vi "FFT_Plugin.vi"(8 "Panel Refs":T1, 9 "Abort VI":refnum<vi>, 10 "Centre VI":refnum<vi>, 11 "Data reference":refnum<vi>) -> ()   [LabVIEW 2016]
uses:
  FFT_Plugin_states.ctl
  <userlib>/Import Export/Excel/Excel.lvclass
  <vilib>/Utility/miscctls.llb/LVMenuShortCut.ctl
  <vilib>/Analysis/baseanly.llb/Mean (DBL).vi
  <userlib>/_OpenG.lib/file/file.llb/Strip Path Extension - String__ogtk.vi
  <vilib>/Analysis/0measdsp.llb/Scaled Time Domain Window (DBL).vi
  <vilib>/Analysis/NI_AALPro.lvlib
  <vilib>/Analysis/NI_AALBase.lvlib
panel:
  in  "Start":dbl=81.44796380090499 format="%#.2g"
  in  "End":dbl=411.76470588235304 format="%#.2g"
  in  "Select data subset manually":bool=TRUE
  in  "Data subset selection":enum32{"Automatic", "Manual"}(radio)
  out "Mean":bool caption="Displaying mean traces"
  in  "Write SD":bool=TRUE caption="Write mean +/-SD"
  in  "Live displays":string="These graphs are live! If you keep this window open, these displays will update as you interact with EMA."
  in  "Frequency display":u16(ring) items=["Log Power Spectrum (dB)", "Power Contribution (RMS)", "Cumulative Power (RMS)"]
  in  "ID":string caption="ID (e.g. name or identifier)"
  in  "Write to Excel":bool
  in  "Inspect":bool
  out "Modifed":cluster{"Time":dbl[], "Data":dbl[]}[](graph)=[{"Time"=[0.0, 4.524886877828055, 9.04977375565611, 13.574660633484164, 18.09954751131222, 22.624434389140276, 27.14932126696833, 31.674208144796385, 36.19909502262444, 40.72398190045249, 45.24886877828055, 49.773755656108605, 54.29864253393666, 58.82352941176472, 63.34841628959277, 67.87330316742083, 72.39819004524888, 76.92307692307693, 81.44796380090499, 85.97285067873305, 90.4977375565611, 95.02262443438916, 99.54751131221721, 104.07239819004526, 108.59728506787332, 113.12217194570138, 117.64705882352943, 122.17194570135749, 126.69683257918554, 131.2217194570136, 135.74660633484166, 140.2714932126697, 144.79638009049776, 149.32126696832583, 153.84615384615387, 158.37104072398193, 162.89592760180997, 167.42081447963804, 171.9457013574661, 176.47058823529414, 180.9954751131222, 185.52036199095025, 190.04524886877832, 194.57013574660638, 199.09502262443442, 203.6199095022625, 208.14479638009053, 212.6696832579186, 217.19457013574663, 221.7194570135747, 226.24434389140276, 230.7692307692308, 235.29411764705887, 239.8190045248869, 244.34389140271497, 248.86877828054304, 253.39366515837108, 257.9185520361991, 262.4434389140272, 266.96832579185525, 271.4932126696833, 276.0180995475114, 280.5429864253394, 285.06787330316746, 289.5927601809955, 294.1176470588236, 298.64253393665166, 303.16742081447967, 307.69230769230774, 312.2171945701358, 316.74208144796387, 321.26696832579194, 325.79185520361995, 330.316742081448, 334.8416289592761, 339.36651583710415, 343.8914027149322, 348.4162895927602, 352.9411764705883, 357.46606334841636, 361.9909502262444, 366.5158371040725, 371.0407239819005, 375.56561085972857, 380.09049773755663, 384.6153846153847, 389.14027149321277, 393.6651583710408, 398.19004524886884, 402.7149321266969, 407.239819004525], "Data"=[0.0, 0.003280547685165013, 0.01289743101562241, 0.02868204224767145, 0.050222095798970356, 0.07622469955534793, 0.10470955152397791, 0.1342620908128156, 0.16506775984322497, 0.1981449543929827, 0.23299766292964016, 0.2662105902390335, 0.2931956236396307, 0.3120584889037999, 0.3258530645330844, 0.3402639325632184, 0.3582301135138749, 0.3764639485856317, 0.3875725425413241, 0.3867580700353336, 0.3767675391078517, 0.3655424378583449, 0.3566337965451223, 0.3388605051396726, 0.282325947397805, 0.14043659443059134, -0.15309830161500587, -0.7030469105570372, -1.6831700852742941, -3.3565583997790314, -6.061772265078592, -10.164326953796436, -16.003914225529716, -23.87323017982634, -34.03144146976264, -46.71611513029193, -62.11103033240042, -80.26582156132996, -101.01544876912169, -123.95678679339927, -148.5001403443597, -173.95829594178113, -199.6215568703556, -224.7966262246939, -248.82566464690345, -271.1095742967033, -291.1362617725535, -308.49403938519396, -322.8603880880117, -333.98337936102394, -341.68028983850377, -345.8596552383632, -346.546630418038, -343.8850717975933, -338.1095786339015, -329.5058674917241, -318.3815784329008, -305.05447076485876, -289.84936776232786, -273.0938258521163, -255.11142903316968, -236.21699940196743, -216.71734765310532, -196.91518147857133, -177.11029181867295, -157.5955080943795, -138.64867636996055, -120.52337364656901, -103.43967106564978, -87.57696817655224, -73.06973510057142, -60.0057900058209, -48.42657074882919, -38.328959252234895, -29.66966154027166, -22.37336695008905, -16.34303372017211, -11.468139565226295, -7.628722188583611, -4.697185233485573, -2.5417035402001376, -1.0322996914069509, -0.047157913061021184, 0.5100193652993072, 0.6618519237579549, 0.7367772454439462, 0.5977863432535553, 0.40162429098039726, 0.17091171829364973, 0.04844407747172897, 0.00765893596057796]}, {"Time"=[0.0, 4.524886877828055, 9.04977375565611, 13.574660633484164, 18.09954751131222, 22.624434389140276, 27.14932126696833, 31.674208144796385, 36.19909502262444, 40.72398190045249, 45.24886877828055, 49.773755656108605, 54.29864253393666, 58.82352941176472, 63.34841628959277, 67.87330316742083, 72.39819004524888, 76.92307692307693, 81.44796380090499, 85.97285067873305, 90.4977375565611, 95.02262443438916, 99.54751131221721, 104.07239819004526, 108.59728506787332, 113.12217194570138, 117.64705882352943, 122.17194570135749, 126.69683257918554, 131.2217194570136, 135.74660633484166, 140.2714932126697, 144.79638009049776, 149.32126696832583, 153.84615384615387, 158.37104072398193, 162.89592760180997, 167.42081447963804, 171.9457013574661, 176.47058823529414, 180.9954751131222, 185.52036199095025, 190.04524886877832, 194.57013574660638, 199.09502262443442, 203.6199095022625, 208.14479638009053, 212.6696832579186, 217.19457013574663, 221.7194570135747, 226.24434389140276, 230.7692307692308, 235.29411764705887, 239.8190045248869, 244.34389140271497, 248.86877828054304, 253.39366515837108, 257.9185520361991, 262.4434389140272, 266.96832579185525, 271.4932126696833, 276.0180995475114, 280.5429864253394, 285.06787330316746, 289.5927601809955, 294.1176470588236, 298.64253393665166, 303.16742081447967, 307.69230769230774, 312.2171945701358, 316.74208144796387, 321.26696832579194, 325.79185520361995, 330.316742081448, 334.8416289592761, 339.36651583710415, 343.8914027149322, 348.4162895927602, 352.9411764705883, 357.46606334841636, 361.9909502262444, 366.5158371040725, 371.0407239819005, 375.56561085972857, 380.09049773755663, 384.6153846153847, 389.14027149321277, 393.6651583710408, 398.19004524886884, 402.7149321266969, 407.239819004525], "Data"=[0.0, 0.0054566161286313305, 0.021176274392851222, 0.046402845232125546, 0.08050972395189936, 0.12246222159496195, 0.1706819140406933, 0.22432346829111416, 0.2842011841463597, 0.3513995755629801, 0.4251048686364699, 0.5014115385742612, 0.5744881966537195, 0.6410198013858962, 0.704505663049861, 0.7729203870067999, 0.8512494069665132, 0.9386660099878618, 1.0317819864568873, 1.1292110414085503, 1.237548340841314, 1.3742350110685522, 1.5563946190062303, 1.781662888227669, 2.013644189539546, 2.1740526496725328, 2.1439449687993104, 1.767900080639427, 0.8400325835065379, -0.9217802670351624, -3.863215671370597, -8.278985381773719, -14.131849697352102, -21.08840503957136, -29.34363717387475, -39.26921136340486, -51.09341268563484, -64.93747332101653, -80.80596778673693, -98.56733824438274, -117.95609965186719, -138.59151554993912, -160.00109682961426, -181.6431484493508, -202.93206429597086, -223.27426115269574, -242.11506061810584, -258.98865795683525, -273.55015617332555, -285.5623040534244, -294.83721215873993, -301.1821976891091, -304.40286334025706, -304.3669529493593, -301.07335219612645, -294.66137882028096, -285.359847882708, -273.4386074364175, -259.20346206447476, -243.01532144426855, -225.29165508030886, -206.4747759908676, -186.99390218825508, -167.25173298757048, -147.63117115923248, -128.49865329528657, -110.19326767484668, -93.00794725153561, -77.17352880118644, -62.85211863155751, -50.1398760216452, -39.073629946225466, -29.63596174019649, -21.75778010787348, -15.324114670246239, -10.18854434827308, -6.192684132978607, -3.18164831793366, -1.0092853331371683, 0.46464487735675375, 1.3769279294274739, 1.8573609250385243, 2.0215250875237833, 1.9543461091327725, 1.5020356466489981, 1.323737337596271, 1.0470392431337219, 0.7219573232570705, 0.38893025356732835, 0.14539394038923847, 0.029094749320411922]}, {"Time"=[0.0, 4.524886877828055, 9.04977375565611, 13.574660633484164, 18.09954751131222, 22.624434389140276, 27.14932126696833, 31.674208144796385, 36.19909502262444, 40.72398190045249, 45.24886877828055, 49.773755656108605, 54.29864253393666, 58.82352941176472, 63.34841628959277, 67.87330316742083, 72.39819004524888, 76.92307692307693, 81.44796380090499, 85.97285067873305, 90.4977375565611, 95.02262443438916, 99.54751131221721, 104.07239819004526, 108.59728506787332, 113.12217194570138, 117.64705882352943, 122.17194570135749, 126.69683257918554, 131.2217194570136, 135.74660633484166, 140.2714932126697, 144.79638009049776, 149.32126696832583, 153.84615384615387, 158.37104072398193, 162.89592760180997, 167.42081447963804, 171.9457013574661, 176.47058823529414, 180.9954751131222, 185.52036199095025, 190.04524886877832, 194.57013574660638, 199.09502262443442, 203.6199095022625, 208.14479638009053, 212.6696832579186, 217.19457013574663, 221.7194570135747, 226.24434389140276, 230.7692307692308, 235.29411764705887, 239.8190045248869, 244.34389140271497, 248.86877828054304, 253.39366515837108, 257.9185520361991, 262.4434389140272, 266.96832579185525, 271.4932126696833, 276.0180995475114, 280.5429864253394, 285.06787330316746, 289.5927601809955, 294.1176470588236, 298.64253393665166, 303.16742081447967, 307.69230769230774, 312.2171945701358, 316.74208144796387, 321.26696832579194, 325.79185520361995, 330.316742081448, 334.8416289592761, 339.36651583710415, 343.8914027149322, 348.4162895927602, 352.9411764705883, 357.46606334841636, 361.9909502262444, 366.5158371040725, 371.0407239819005, 375.56561085972857, 380.09049773755663, 384.6153846153847, 389.14027149321277, 393.6651583710408, 398.19004524886884, 402.7149321266969, 407.239819004525], "Data"=[0.0, 0.0011044792416986951, 0.004618587638393602, 0.010961239263217359, 0.019934467646041367, 0.02998717751573392, 0.03873718900726252, 0.04420071333451705, 0.0459343355400902, 0.044890333222985246, 0.040890457222810414, 0.03100964190380573, 0.011903050625541855, -0.01690282357829643, -0.052799533983692234, -0.09239252188036301, -0.13478917993876346, -0.18573811281659838, -0.25663690137423906, -0.3556949013378831, -0.4840132626256104, -0.6431501353518624, -0.8431270259159858, -1.103941877948324, -1.4489922947439358, -1.8931794608113501, -2.450141572029322, -3.1739939017535015, -4.206372754055126, -5.7913365325229, -8.260328858786588, -12.049668525819156, -17.87597875370733, -26.658055320081328, -38.719245765650534, -54.163018897179, -73.12864797916599, -95.59416980164337, -121.22492975150645, -149.34623534241578, -179.0441810368522, -209.32507633362317, -239.24201691109693, -267.950104000037, -294.71926499783604, -318.94488744071083, -340.1574629270011, -357.9994208135527, -372.1706200026979, -382.4044546686235, -388.5233675182676, -390.5371127876173, -388.69039749581884, -383.4031906458273, -375.1458050716765, -364.35035616316725, -351.4033089830936, -336.6703340933, -320.49527346018095, -303.17233025996404, -284.9312029860305, -265.95922281306724, -246.44079311795556, -226.57862996957223, -206.5894124781134, -186.69236289347248, -167.1040850650744, -148.03880004160243, -129.70581333011313, -112.30181772154698, -95.99959417949765, -80.93795006541633, -67.2171797574619, -54.90013839659631, -44.01520841029709, -34.558189551905016, -26.493383307365608, -19.754630812518933, -14.248159044030054, -9.8590153443279, -6.460335009827748, -3.9219603078524257, -2.1158409136458256, -0.9343073785341579, -0.17833179913308825, 0.14981715329162126, 0.14853344337338872, 0.08129125870372385, -0.04710681698002889, -0.04850578544578052, -0.013776877399256001]}] caption="XY Graph"
  in  "Abort":bool=TRUE
  in  "Periodic extension (zero padding)":bool
  in  "Remove DC Component":bool
  in  "Apply window":bool=TRUE
  in  "Window":u16(ring)=1 items=["Rectangle", "Hanning", "Hamming", "Blackman-Harris", "Exact Blackman", "Blackman", "Flat Top", "4 Term B-Harris ", "7 Term B-Harris", "Low Sidelobe", "Blackman Nuttall", "Triangle", "Bartlett-Hanning", "Bohman", "Parzen", "Welch", "Kaiser", "Dolph-Chebyshev", "Gaussian"]
  in  "stop":bool=TRUE
  in  "Live data":cluster{dbl, dbl, "Impulses":dbl[][]}(graph)={0.0, 4.524886877828055, "Impulses"=[[1.410730292612453, 1.3768034370367894, 1.3548353514357787, 1.341757359189093, 1.3252268542692756, 1.2918927209333702, 1.23781873081185, 1.1721445111231026, 1.1099562251709596, 1.0599166586354007, 1.0172490394533225, 0.9686595339431536, 0.9047673910478693, 0.8288181580322441, 0.7544025685957787, 0.694320690605783, 0.6505827404540062, 0.6137999925050119, 0.571742484121512, 0.519863429471382, 0.46442129820892636, 0.4156426193698084, 0.3761013091270612, 0.33311079925207554, 0.25992068556340814, 0.12161862542107932, -0.1252316400992416, -0.5453137519834004, -1.2425542690526563, -2.366660512170925, -4.095965103495613, -6.603127826568753, -10.026682854478048, -14.467711625845375, -20.006989082761383, -26.71765968791203, -34.650952736880704, -43.79728933083065, -54.05109908114851, -65.20716298219895, -76.99269469879322, -89.11260780001447, -101.28231848622046, -113.23974163442473, -124.7470593418671, -135.59518498445283, -145.61151288418924, -154.66139432364216, -162.6386816612302, -169.4536979266029, -175.03058130417614, -179.31745237847906, -182.3000030507743, -184.00518252156053, -184.4905185408141, -183.8271266774419, -182.08728700462382, -179.3406685891595, -175.65520191995512, -171.09721676508144, -165.72994784425535, -159.61282346036108, -152.804250039799, -145.3672457276378, -137.37444300835176, -128.91027361336867, -120.07028157394262, -110.95869222566036, -101.68453089228515, -92.35751827130296, -83.08446010208225, -73.96594451991314, -65.0928968197739, -56.542432632023775, -48.37445417938233, -40.632336128292174, -33.34854321380435, -26.550598679863526, -20.261661506765652, -14.494964066015047, -9.248487689619074, -4.506937349962988, -0.2522570296729517, 3.4294956811031243, 5.778147017617445, 8.70977538890169, 10.131569294830525, 10.597791415646018, 7.995318248677886, 5.088900932820739, 3.214356371728213, 1.4314128213908817], [2.364341969813819, 2.2900712202609257, 2.2245023155686567, 2.170743580247381, 2.124436396241567, 2.0755483929849197, 2.01770771754292, 1.9584047923111045, 1.9110386779575452, 1.8797060218748745, 1.855973634456436, 1.8244843934756714, 1.7728033605066527, 1.702529717788376, 1.6310446015189317, 1.5771716174771009, 1.5459564986366559, 1.5304339022630353, 1.522072725122912, 1.5178365238247493, 1.5254599916191358, 1.5625836578011185, 1.6413532856314563, 1.7514320485671622, 1.8538422807040986, 1.8827378712669303, 1.7537081854795642, 1.3712601700239306, 0.6201310740437038, -0.6499338605382539, -2.610391134020305, -5.378339264237013, -8.853807453958103, -12.780045283497623, -17.251042072603628, -22.458661695090797, -28.504364179132295, -35.43332955585003, -43.23745946198392, -51.851105985309815, -61.15656151769813, -70.99547223516495, -81.18002034102021, -91.5014764479077, -101.73861407351457, -111.6704005080021, -121.09360769422771, -129.84220710857412, -137.79899427032026, -144.88621710119986, -151.034549457443, -156.15358303107433, -160.13037797728035, -162.85992421311624, -164.28158909283007, -164.38783024920167, -163.2016549976529, -160.7537911271449, -157.08309739913255, -152.2526003678371, -146.3579048093173, -139.51587757309167, -131.84668092020377, -123.46901638065522, -114.5091552863219, -105.10957295384713, -95.42778931381324, -85.62687785264612, -75.8640663935449, -66.28301727917503, -57.01190134479019, -48.1639845840505, -39.83537487539351, -32.09682287160172, -24.98497267821006, -18.50344472249384, -12.63639284811454, -7.366030658195303, -2.6806321266190096, 1.433839728680736, 5.010222790892419, 8.109088276495406, 10.813538617119217, 13.141504022534892, 13.11317906694486, 15.648494786805148, 17.745722641436604, 19.050523822150993, 18.194312156332213, 15.27318503082378, 12.21069001533261, 7.3082855694758475], [0.4571186154110868, 0.46353565381265327, 0.4851683873029008, 0.512771138130805, 0.5260173122969842, 0.5082370488818209, 0.4579297440807799, 0.3858842299351005, 0.30887377238437397, 0.24012729539592703, 0.17852444445020899, 0.11283467441063588, 0.03673142158908582, -0.04489340172388767, -0.1222394643273742, -0.18853023626553478, -0.24479101772864342, -0.30283391725301145, -0.3785877568798881, -0.47810966488198536, -0.596617395201283, -0.7312984190615017, -0.8891506673773341, -1.0852104500630113, -1.3340009095772822, -1.6395006204247715, -2.004171465678047, -2.4618876739907316, -3.1052396121490164, -4.083387163803597, -5.58153907297092, -7.827916388900492, -11.199558254997994, -16.15537796819313, -22.762936092919137, -30.97665768073326, -40.79754129462911, -52.16124910581127, -64.8647387003131, -78.56321997908809, -92.82882787988831, -107.22974336486399, -121.38461663142071, -134.97800682094174, -147.75550461021965, -159.51996946090355, -170.12941807415075, -179.4805815387102, -187.47836905214015, -194.02117875200594, -199.02661315090927, -202.4813217258838, -204.46962812426827, -205.1504408300048, -204.6994479887981, -203.26642310568212, -200.97291901159474, -197.9275460511741, -194.22730644077768, -189.9418331623258, -185.1019908791934, -179.7097693476305, -173.76181915939424, -167.26547507462038, -160.2397307303816, -152.7109742728902, -144.712773834072, -136.2905065986746, -127.5049953910254, -118.4320192634309, -109.1570188593743, -99.76790445577578, -90.35041876415428, -80.98804239244583, -71.76393568055461, -62.76122753409051, -54.060693579494156, -45.73516670153175, -37.842690886912294, -30.423767860710832, -23.507198170130565, -17.12296297642138, -11.318052676465122, -6.282512660328643, -1.5568850317099683, 1.7710559909982306, 2.517415948224447, 2.1450590091410415, -2.20367565897644, -5.095383165182303, -5.781977271876183, -4.445459926694085], [0.5023568318808596, 0.4893032590680133, 0.49512843757511926, 0.500047627047562, 0.48387712339247213, 0.4463428139727666, 0.4105470731967099, 0.40463061098914344, 0.4376463080092003, 0.4918853432629796, 0.5385413016613759, 0.5616941128357155, 0.5692138239041419, 0.5821157750397432, 0.6149119682566897, 0.6655257740297786, 0.7208605817914435, 0.7698018741854714, 0.8103861925510321, 0.8474898436816303, 0.887864780805265, 0.9375185517498736, 1.0001445273795566, 1.0738398057046237, 1.149548314048465, 1.2179439408484987, 1.285144372535588, 1.3833571315004367, 1.55999092462304, 1.8436470995521317, 2.2106634093212976, 2.5828681847113555, 2.8655582613049986, 3.0017191555559726, 3.003243389547119, 2.9394601145426895, 2.899301727675939, 2.960927470291303, 3.187483759635348, 3.6357361507565598, 4.35242738097167, 5.351830664232269, 6.594802226039589, 7.9950808295073745, 9.4553018038476, 10.907483107105017, 12.32874338057431, 13.725053926941623, 15.099607683510994, 16.430135556602362, 17.66711227556626, 18.749505584342824, 19.626001891778035, 20.269644324484567, 20.678235309300817, 20.861161720497595, 20.823903454212292, 20.565781901123675, 20.09654832301661, 19.45749107439412, 18.72273690523542, 17.971852691824232, 17.251893874532406, 16.561074428958364, 15.868972337133066, 15.154425182879812, 14.427593002881142, 13.718510695871757, 13.045049915207473, 12.391027427844957, 11.713505451661385, 10.973422679301992, 10.166330988933517, 9.33132231376839, 8.53068543424369, 7.812179601817312, 7.177734260878598, 6.582336612566129, 5.9675827457377215, 5.306315108243301, 4.622820187801937, 3.9689980802963487, 3.376119088371326, 2.8823122355666553, 2.2903695084639235, 1.74682508021205, 1.087631196240318, 0.6199203351200653, 0.2799378552104854, 0.16439572434565985, 0.0984395550677905, 0.13231348780272795], [1.2806770464228152, 1.2819836526066268, 1.3057566437960637, 1.3078837401439865, 1.2635371713360157, 1.188015892586324, 1.1197640828738749, 1.0930985125685955, 1.1147036889851334, 1.1591139554508967, 1.1955980114109348, 1.2084889615010135, 1.1996192567179116, 1.1922705220673417, 1.2097121688099948, 1.2472776797782872, 1.2959433980469712, 1.355528349106264, 1.4105906990562982, 1.4493738626633803, 1.4827087235283551, 1.5235075063052412, 1.58268412391006, 1.6682273812114417, 1.76940993451494, 1.8699579946172311, 1.9759712136701804, 2.120593404919596, 2.3439389358508866, 2.6634060822558356, 3.0593535489211616, 3.473113221158675, 3.8150646225118967, 4.011252980545241, 4.070742022765055, 4.104461153750526, 4.2504728044926585, 4.576307211048022, 5.10283115778458, 5.8772169708494, 6.96669915513311, 8.395206659253137, 10.102375743870343, 11.967375447685601, 13.869958419320628, 15.725982547852617, 17.492807941831806, 19.179160195859225, 20.82597706014503, 22.429034114548333, 23.8931934945146, 25.09384321384666, 25.964849305648727, 26.51429989736166, 26.783843727193812, 26.817608056436, 26.65181277982765, 26.30940823133898, 25.804911564823364, 25.145509892363634, 24.33126903352085, 23.393061077570334, 22.421743479829725, 21.50330731642481, 20.626636229942143, 19.718396527916962, 18.74988133125357, 17.76195064348292, 16.827954501857313, 15.991592772861058, 15.2000443824661, 14.361934988791564, 13.47627515294208, 12.61968455014931, 11.846212531594242, 11.158577412867583, 10.527352100572394, 9.922823291343615, 9.335625633440277, 8.742743856118311, 8.0981342384547, 7.387103058776486, 6.649124875775302, 5.929925072660412, 5.229415266600543, 4.553123721380457, 3.703916334369808, 2.9664692085587516, 2.100478303350439, 1.0767837594622454, 0.8247909324752697, 0.7200327482509221], [-0.275963382661096, -0.3033771344706002, -0.3154997686458252, -0.30778848604886244, -0.29578292455107147, -0.29533026464079076, -0.29866993648045503, -0.2838372905903087, -0.23941107296673275, -0.17534326892493757, -0.11851540808818284, -0.08510073582958244, -0.061191608909627715, -0.02803897198785532, 0.02011176770338463, 0.08377386828127009, 0.1457777655359157, 0.18407539926467886, 0.21018168604576604, 0.24560582469988013, 0.2930208380821747, 0.35152959719450594, 0.41760493084905337, 0.4794522301978057, 0.5296866935819898, 0.5659298870797661, 0.5943175314009956, 0.6461208580812772, 0.776042913395193, 1.0238881168484277, 1.3619732697214335, 1.6926231482640357, 1.9160519000981007, 1.9921853305667037, 1.9357447563291825, 1.7744590753348528, 1.5481306508592194, 1.345547729534585, 1.2721363614861152, 1.3942553306637193, 1.7381556068102295, 2.308454669211401, 3.0872287082088357, 4.022786211329148, 5.040645188374573, 6.088983666357419, 7.164678819316811, 8.27094765802402, 9.37323830687696, 10.431236998656392, 11.441031056617923, 12.405167954838989, 13.287154477907341, 14.024988751607474, 14.572626891407822, 14.90471538455919, 14.995994128596935, 14.822155570908368, 14.388185081209857, 13.769472256424608, 13.114204776949986, 12.55064430607813, 12.082044269235087, 11.618841541491916, 11.111308444323988, 10.590453837842663, 10.105304674508714, 9.675070748260595, 9.262145328557631, 8.790462082828856, 8.22696652085667, 7.58491036981242, 6.856386824924953, 6.042960077387468, 5.215158336893138, 4.465781790767041, 3.828116421184802, 3.241849933788643, 2.5995398580351656, 1.8698863603682905, 1.1475061371491733, 0.5508931018162122, 0.10311330096735061, -0.1653006015271017, -0.6486762496726959, -1.0594735609563568, -1.5286539418891716, -1.7266285383186208, -1.5406025929294682, -0.7479923107709258, -0.6279118223396888, -0.45540577264546617], [0.1428609168455076, 0.14009219140856577, 0.11947094183009842, 0.10077072367996759, 0.10664090057570925, 0.1408336768786598, 0.18290439134056327, 0.20532583194411785, 0.19704920610655483, 0.17131130147226892, 0.1509822095157714, 0.1472165016489006, 0.15162634039696785, 0.14726502462371371, 0.12541493294154754, 0.09187568505023, 0.059738087262853436, 0.03763662423540375, 0.024354767043458726, 0.011872031120744184, -0.00918999562797793, -0.0452084842455664, -0.09561082366349702, -0.1497420825160259, -0.1891829523968459, -0.19914511043679145, -0.18438773967785893, -0.17412197827471515, -0.2042001861453794, -0.28370161023986207, -0.3747421958073463, -0.41126283022121707, -0.3532835017017899, -0.2380282980415485, -0.18401709146102072, -0.3383244204315349, -0.8030823749571163, -1.5930376472087437, -2.6484391507481364, -3.88027583371108, -5.2058441553407535, -6.553143684831892, -7.848861818194611, -9.01821298931344, -10.00567137165893, -10.79874350413909, -11.430302235646876, -11.95285993523213, -12.400011764816897, -12.759417712509943, -12.972360283883038, -12.96031169842876, -12.664019458488333, -12.071631899296586, -11.216711005472934, -10.14751511736184, -8.893711046765965, -7.462892813463602, -5.872300712223161, -4.184494771149863, -2.5064055575799684, -0.9440319396179457, 0.45049034184902637, 1.6921303705819244, 2.825883972816616, 3.87539217302074, 4.82232194829527, 5.629306467522421, 6.279705590623783, 6.796762560700551, 7.229567603800389, 7.6216667224063706, 7.986642529547609, 8.304001897706291, 8.535683828129462, 8.652899248132748, 8.658862383256903, 8.591141998324726, 8.497475232866881, 8.400366725850619, 8.279505830654616, 8.090912186563397, 7.808832818723973, 7.241765629335075, 6.764355433821842, 6.380256170327707, 5.610727778846916, 4.487705481763241, 2.3698890985403973, 1.046250262014416, 0.42115130680965274, 0.0698224820121571], [0.7895528092077438, 0.7889645815842736, 0.7864982274026173, 0.7729337942321055, 0.7600503286681314, 0.7669180118298423, 0.7893386673117864, 0.8006965234119674, 0.7842792421592614, 0.7493836302729078, 0.7189433695337686, 0.7060017388053474, 0.70276193720043, 0.6950077931420253, 0.6718222239528342, 0.627505042151405, 0.5768263030203996, 0.5455471491014274, 0.534831905263048, 0.5224517112206513, 0.49008901261597826, 0.43575610802911896, 0.3724430942425503, 0.316782300810857, 0.2902199423782129, 0.3120135773721317, 0.3700048441619669, 0.42741629635065864, 0.4514998031343632, 0.4382643470086537, 0.4390392345620275, 0.5309452349275028, 0.7486940203525712, 1.0750380030480298, 1.4611155862724352, 1.813727417358169, 2.000364202769248, 1.9140182677827258, 1.537245321751846, 0.954703019325799, 0.29623030530770667, -0.3512896640963268, -0.9703807431636662, -1.5589288536235344, -2.084259572863407, -2.5012370465985505, -2.7939964423148, -2.9808859933857335, -3.0964144401108022, -3.1865081450918087, -3.287512379703312, -3.3729256937246923, -3.3334063465379735, -3.040229895146185, -2.439124577777161, -1.574064829191606, -0.5235420399304385, 0.6653420228090638, 1.9710431349929163, 3.3341480502154575, 4.625873721771791, 5.7140661618930295, 6.5669030810059645, 7.268357929590209, 7.922340404082234, 8.562022331023298, 9.146307556723766, 9.609889191511309, 9.938233958837124, 10.205346009285696, 10.503607392913068, 10.880846490462496, 11.349120062138814, 11.847728145359298, 12.248885237974134, 12.459822111756324, 12.473877235002584, 12.361579285203078, 12.228256884357315, 12.111771330098415, 11.943313468034535, 11.649768995915846, 11.23741208771981, 10.810655788857671, 10.350963760424722, 9.800349076558891, 9.259991702318938, 8.304543842410949, 5.751621749962787, 3.4052503349066274, 1.885089117525665, 0.5426199180611824], [-0.5038309755167286, -0.5087801987671421, -0.5475563437424205, -0.5713923468721704, -0.5467685275167128, -0.48525065807252277, -0.4235298846306599, -0.39004485952373164, -0.39018082994615166, -0.40676102732836994, -0.41697895050222583, -0.4115687355075463, -0.39950925640649426, -0.4004777438945979, -0.42099235806973906, -0.44375367205094496, -0.4573501284946927, -0.47027390063061997, -0.48612237117613055, -0.49870764897916287, -0.5084690038719342, -0.5261730765202518, -0.5636647415695444, -0.6162664658429088, -0.6685858471719047, -0.7103037982457145, -0.7387803235176847, -0.7756602529000889, -0.859900175425122, -1.005667567488378, -1.18852362617672, -1.3534708953699368, -1.455261023756151, -1.5510945991311267, -1.8291497691944765, -2.490376258221239, -3.6065289526834805, -5.100093562200213, -6.834123623248119, -8.715254686747958, -10.707918615989215, -12.754997705567458, -14.727342893225556, -16.477497125003346, -17.927083170454456, -19.09624996167963, -20.06660802897895, -20.924833877078527, -21.703609089522992, -22.33232727992808, -22.657208188062764, -22.547697703132826, -21.994632570438693, -21.103033903446985, -19.994297433168708, -18.720965405532073, -17.26388005360149, -15.591127649736269, -13.715644559439239, -11.703137592515183, -9.638684836931727, -7.602130041128921, -5.665922397307911, -3.88409718842636, -2.270572458449002, -0.8112379849818177, 0.4983363398667757, 1.6487237435335342, 2.6211772224104406, 3.388179112115406, 3.955527814687709, 4.362486954350246, 4.624164996956404, 4.760275650053283, 4.822482418284791, 4.8459763845091715, 4.843847531511221, 4.820704711446375, 4.7666935813764475, 4.688962121602822, 4.615698193274695, 4.532055377210948, 4.3802535497281365, 3.6728754698124786, 3.177747107218962, 2.9601632640965225, 1.9614638553748929, 0.6708671211155335, -1.0118435528819925, -1.3127498108777953, -1.0427865039063593, -0.4029749540368681], [0.8533007616422014, 0.8320714964959047, 0.8196882933654313, 0.8079448596831116, 0.7909464909994228, 0.7720577378667189, 0.7635056302479306, 0.777559929756277, 0.8159745504156796, 0.8669422250473191, 0.9125946222233504, 0.9415719339262932, 0.9566162500524569, 0.9705010485562443, 0.9950317781156892, 1.033071260791991, 1.0791888986124714, 1.126300875048726, 1.1704139113090224, 1.2104036620287582, 1.2464404189402403, 1.2806429666154864, 1.3188071312898992, 1.3688967345275418, 1.4365238639336193, 1.5232877289212883, 1.6330808615694297, 1.7822404386987416, 2.001960136635468, 2.323609122176582, 2.7516079794967765, 3.2414643864195596, 3.6992278552060047, 4.007043642180823, 4.063210441143857, 3.818699939609508, 3.297149449733941, 2.5943461384802746, 1.859343611972152, 1.2614315398989966, 0.9494176760733919, 1.0154878240495895, 1.4775969310388501, 2.2885387520450227, 3.366144675673136, 4.626767037284251, 6.0051738601788385, 7.4572974725508185, 8.954058207717338, 10.476302823265534, 12.012709504190957, 13.555493386738936, 15.09133859202418, 16.59397400886831, 18.026729814882497, 19.354622714624302, 20.555735639729008, 21.621514871912634, 22.548510483073205, 23.332552996011753, 23.97154289854723, 24.472005878131295, 24.848352635834072, 25.113026435485096, 25.26799987291367, 25.306985796617738, 25.22601964536895, 25.030210349184628, 24.72819210254418, 24.3203216008959, 23.794965876471103, 23.140429901127757, 22.364005693671263, 21.500484468712234, 20.599894865575504, 19.700989592717224, 18.809711522101438, 17.899971707920724, 16.936911686472836, 15.904629518153554, 14.81716083665625, 13.703923100751274, 12.583386221685391, 11.317970683867356, 10.00342705553732, 8.850639889857053, 7.148870567430042, 5.36440522728091, 2.7657810100007008, 1.2787409249801975, 0.5603658606604953, 0.25694201094766267], [1.5756044428356446, 1.5430067625100912, 1.5252045261135034, 1.5092660936195208, 1.4835766061817832, 1.4478712367684148, 1.4168706830915894, 1.413345866123949, 1.4446614641472526, 1.49352412873363, 1.536466401015578, 1.5598875127117107, 1.5651397159981455, 1.5679944669255153, 1.5841381298942583, 1.6143550927415997, 1.6538353290681425, 1.7025283705373409, 1.755045328634939, 1.8032435899676944, 1.8476868554787071, 1.8908487046295532, 1.9365519425045128, 1.9975252455999897, 2.083885944833346, 2.1926306019069823, 2.3226303850165424, 2.4929140255467996, 2.7385391000381527, 3.0887982428339598, 3.5526226280568594, 4.11670909190989, 4.743993660945112, 5.3761892288248205, 5.943019533553599, 6.369635184996055, 6.594108333229062, 6.604955076530372, 6.474899468154027, 6.351842132618369, 6.400966142676911, 6.744519893206698, 7.437302873617837, 8.466845374653317, 9.762592408548993, 11.219659404281234, 12.735241308194377, 14.240715961567727, 15.71365830661301, 17.16737184021246, 18.628258131124745, 20.1088018919615, 21.58160862283678, 22.97562649993662, 24.210350214230214, 25.244805687567602, 26.09479781317968, 26.80346860997333, 27.40494548219024, 27.90911231545381, 28.303126656279794, 28.588313487252584, 28.81694974004713, 29.037816850709437, 29.21783520920017, 29.28273964522523, 29.203479766937182, 29.007387928683162, 28.731646497562927, 28.373739765747175, 27.88610416625275, 27.226070296868453, 26.406161410113874, 25.495359035001943, 24.5752414096585, 23.690130134772676, 22.833212330921462, 21.967321157506376, 21.050768666311708, 20.057121515396126, 18.983215634368655, 17.839769830829805, 16.643097895977448, 15.585359402191163, 14.41353444519629, 13.039368118577533, 11.564001575813588, 9.833831106825002, 6.67662681422695, 4.198669954222929, 2.1125273214943396, 1.2679975953042555], [0.13099708044875813, 0.1211362304817184, 0.11417206061735918, 0.10662362574670248, 0.09831637581706232, 0.09624423896502321, 0.11014057740427174, 0.14177399338860497, 0.18728763668410653, 0.24036032136100816, 0.28872284343112276, 0.3232563551408757, 0.34809278410676814, 0.37300763018697347, 0.40592542633712025, 0.4517874288423822, 0.5045424681568003, 0.550073379560111, 0.5857824939831058, 0.6175637340898219, 0.6451939824017734, 0.6704372286014195, 0.7010623200752858, 0.7402682234550938, 0.7891617830338923, 0.853944855935594, 0.943531338122317, 1.0715668518506836, 1.2653811732327829, 1.5584200015192042, 1.9505933309366936, 2.3662196809292295, 2.6544620494668973, 2.637898055536825, 2.1834013487341153, 1.2677646942229615, 0.00019056623881974488, -1.416262799569823, -2.756212244209723, -3.828979052820376, -4.502130790530128, -4.713544245107519, -4.482109011540135, -3.889767870563272, -3.030303057202722, -1.9661253297127317, -0.7248935878367, 0.6738789835339114, 2.1944581088216673, 3.78523380631861, 5.397160877257166, 7.002184881516372, 8.60106856121158, 10.212321517800003, 11.84310941553478, 13.464439741681002, 15.016673466278334, 16.43956113385194, 17.69207548395617, 18.755993676569695, 19.639959140814668, 20.355698269010006, 20.879755531621015, 21.188236020260756, 21.31816453662717, 21.331231948010245, 21.24855952380072, 21.053032769686094, 20.724737707525435, 20.266903436044622, 19.703827586689457, 19.05478950538706, 18.321849977228652, 17.505609902422524, 16.624548321492508, 15.711849050661773, 14.786210713281415, 13.83262225833507, 12.823054706633965, 11.75213752091098, 10.651106038943842, 9.568076370672742, 8.523674547393334, 7.05058196554355, 5.593319665878351, 4.661911661136573, 2.733739559046496, 0.8949793477368191, -1.1450647942255476, -1.641188104262534, -0.9917956001733492, -0.75411357340893], [2.2825610735445365, 1.6193230987095557, -1.2849820096799227, -4.320985047234379, -5.381459413060144, -4.176678713666436, -2.2882677530372515, -1.4904682232865523, -2.082428596286533, -2.854711803833296, -2.5515901864208974, -1.2330459814903496, -0.1952032354127965, -0.6387397674322222, -2.4710664162134135, -4.373059705639674, -4.970109636560661, -3.9761352472064044, -2.358589667102657, -1.4915748039657968, -2.0240172303013564, -3.334905748584171, -3.943125994157051, -2.59776279122075, 0.673805767698131, 4.420827434851322, 6.73737934298327, 6.66096186239298, 4.931261250610796, 3.446973885506109, 3.8746207505011148, 6.60264779986794, 10.847583718022422, 15.682044284208619, 20.964630804484898, 27.377257768501018, 35.75421884997374, 46.385669442385655, 58.79854550912392, 72.05157168374596, 85.24788809630584, 97.96181470436719, 110.36678021867398, 122.9565320416245, 135.96202963453283, 148.91112895943164, 160.82243042909846, 170.9642555285605, 179.44688998924005, 186.97120397453466, 193.91619456235878, 199.76175924005014, 203.59875464326404, 205.30018492540896, 206.0660271446944, 207.56317264519944, 210.3530823047164, 213.14734435130453, 213.71207601600776, 210.62498682422188, 204.28124128150628, 196.34608236643365, 188.3259176594273, 180.58796550691932, 172.50215221488756, 163.2571191835404, 152.49349289314904, 140.41009768840135, 127.57536538807628, 114.74636441393602, 102.67447441726486, 91.77285697713005, 81.86518265971054, 72.32320072168578, 62.60998857207962, 52.78974965415986, 43.45912169914968, 35.14887122859104, 27.82585939558083, 21.021946002791335, 14.435387239341427, 8.278363206656431, 2.9496253155434617, -1.3483760411605146, -4.160633670200097, -8.532165813134927, -11.373486399666636, -12.953226674643206, -10.198865386599625, -6.054972325489615, -3.886647748801941, -1.784995149317917], [31.6011387585613, 30.682176150333987, 17.13159058407684, 1.2606610189742007, 3.199298818738791, 8.431102090258182, 11.584523356481265, 11.346477745042716, 5.412579330152584, 2.0426748197454945, 11.896811492467464, 19.795470556122773, 20.2512474096065, 12.198745989097235, 1.0932285970344608, 1.830844124150338, 2.1780985391629253, -0.18461438053893042, 0.6658550416306879, 2.8643870458147482, 1.1631486547555325, 0.8057697554662275, 0.920369029296829, 1.4006393504641963, 17.823018782793266, 37.64837695486858, 49.672791208536836, 47.67975390494491, 34.15004911799332, 18.02334692906269, 8.517823974998423, 10.287150265764708, 14.683787746237256, 19.099861478361877, 24.629592912147448, 32.857133591546486, 43.16485429408401, 55.077675595207964, 69.03638739879156, 84.41392008040003, 100.54709162702244, 116.76094032880908, 130.63564324377433, 142.12937699804502, 155.4485930268446, 170.1061977896586, 182.00801734225274, 193.2831591404493, 204.30183877060807, 210.38851372249607, 212.73377704600048, 219.33484458227548, 228.7608321437212, 233.5317756318039, 233.3692916663306, 232.57719789614282, 234.2125372684578, 236.8057562757666, 237.51493955512007, 234.02289398738714, 226.22074703613265, 218.6461915562746, 214.28521323115413, 209.9594073899002, 202.79028140235388, 192.68543931215274, 181.1818595335017, 169.38570205611688, 156.98426361922046, 144.4142980757566, 133.15400009887, 123.33111052541403, 113.9736356053802, 104.071275964053, 92.54805570898645, 79.45793385574865, 66.75233055443037, 56.29128406978212, 47.78336374406572, 39.90741667429724, 32.041662925717226, 24.35017614741126, 17.28310909513854, 11.465912730521428, 5.75214178300728, 1.230524599838514, -1.5725452100641437, -2.4307882394015685, 2.583141530894702, 6.245604974146939, 7.262335553144695, 5.654160758145034], [-27.03601661147223, -27.443529952914872, -19.701554603436684, -9.90263111344296, -13.962217644859079, -16.784459517591053, -16.16105886255577, -14.32741419161582, -9.577436522725652, -7.752098427412086, -16.99999186530926, -22.26156251910347, -20.641653880432095, -13.476225523961679, -6.035361429461288, -10.576963535429687, -12.118317812284246, -7.767656113873878, -5.383034375836002, -5.847536653746342, -5.211183115358246, -7.475581252634569, -8.806621017610931, -6.596164932905697, -16.475407247397005, -28.806722085165934, -36.1980325225703, -34.35783018015895, -24.287526616771725, -11.129399158050472, -0.7685824739961937, 2.9181453339711707, 7.011379689807589, 12.26422709005536, 17.299668696822348, 21.89738194545555, 28.343583405863466, 37.69366328956335, 48.560703619456284, 59.689223287091885, 69.94868456558925, 79.16268907992529, 90.09791719357362, 103.78368708520398, 116.47546624222105, 127.71606012920466, 139.63684351594418, 148.6453519166717, 154.59194120787203, 163.55389422657325, 175.09861207871708, 180.1886738978248, 178.4366771428069, 177.06859421901402, 178.7627626230582, 182.54914739425607, 186.493627340975, 189.48893242684244, 189.90921247689545, 187.22707966105662, 182.34173552687992, 174.0459731765927, 162.36662208770045, 151.21652362393843, 142.21402302742123, 133.82879905492806, 123.80512625279638, 111.4344933206858, 98.16646715693211, 85.07843075211545, 72.19494873565972, 60.21460342884606, 49.756729714040894, 40.575125479318565, 32.67192143517279, 26.12156545257108, 20.165912843868984, 14.006458387399963, 7.868355047095946, 2.1364753312854283, -3.170888447034372, -7.793449734098397, -11.383858464051617, -14.162664812842458, -14.073409123407474, -18.29485622610837, -21.17442758926913, -23.475665109884844, -22.98087230409395, -18.35554962512617, -15.035631050748577, -9.224151056780869], [-1.1981496477847582, -1.2478607091493559, -0.4972677927914925, 0.48005669892835245, 0.9959155512020954, 0.8227865344808531, 0.3538789450461943, 0.21056821192052508, 0.6542991333536923, 1.3525947019277265, 1.7145571624058944, 1.4472378634972867, 0.7832176592562639, 0.21888209791481628, 0.06259045619102394, 0.21990210358044887, 0.37377939670868654, 0.32318337599716396, 0.13181950738229678, -0.023701809606681723, -0.1005349069863002, -0.2592791153907109, -0.6689045311506439, -1.2444037388538263, -1.6224847522755697, -1.454289061786538, -0.791956150702996, -0.16828101558650402, -0.21104429464687258, -1.1239503660837502, -2.5201351335908626, -3.8036015331879853, -4.71483145078048, -5.452503521473123, -6.266936347855861, -7.04741605981341, -7.4503168125285235, -7.4282991364178725, -7.47044307479012, -8.129168111493136, -9.294778938885578, -10.115818528923805, -9.777712059859862, -8.33733920998134, -6.711530577346904, -5.8253823699826945, -5.854541726763927, -6.368658414108912, -7.075469803911694, -8.161600360867117, -9.774999340336551, -11.314683449277194, -11.551784176655634, -9.656484357429928, -6.092248938727362, -2.348018210481238, 0.33705660647427077, 2.008211503933337, 3.784312202061498, 6.665129866451432, 10.588256817764439, 14.569430928598218, 17.601892599428272, 19.35389261689661, 20.096018051074694, 20.176087972546274, 19.704184729852802, 18.67882384855385, 17.235221491711428, 15.67213657222401, 14.264144586499325, 13.099833463192951, 12.103687960677084, 11.145020390079699, 10.089057642000226, 8.807038222252451, 7.226045693098076, 5.42288717698219, 3.611021530002709, 1.9792553203757457, 0.5694983982567897, -0.6713215729586242, -1.7264661920179507, -2.427965711465797, -2.435216619568162, -2.579862187134526, -2.514457039007956, -2.782504686644563, -2.561875575189057, -2.0441084796839446, -1.362531396536606, -0.5852815158377919], [4.515475527764445, 6.6934451589817225, 7.487855134636235, 6.970868492876893, 6.0932797582553375, 4.693232105536136, 4.374886001478088, 4.906655003012542, 4.502308274827208, 4.861192620635503, 6.536753395251109, 6.431218471709848, 4.944409250799032, 3.9873332498503453, 3.547881596710193, 3.5159753484095813, 4.0484703294828135, 4.2843880036256206, 3.833157178924912, 3.0841172462458277, 3.0328961720500502, 3.4845787294685917, 3.1580437906241023, 2.3446760007881013, 2.7308431649357097, 4.3260954389714, 5.4002175065755464, 4.791733616623865, 3.866209229206044, 4.30135767132807, 3.3925116422451422, 0.7293104865251281, -0.7628452447355181, -0.5353460304838231, -1.5109182289741288, -2.523454248055545, -1.8944879891757145, -1.1856612719251869, -0.675360685773847, -0.5733749336038345, -1.4517410123473748, -1.648138146328554, -0.4822346477503121, 0.7582760046303143, 2.491907642879246, 4.145024303858277, 3.697943685123711, 4.5147229440079695, 7.856564242441199, 7.9332701405633745, 3.3639403855602126, 0.30460651211483736, 1.737309504643017, 3.585739958024046, 6.557559267408287, 11.18808503520422, 14.080574535276352, 15.803534784828983, 18.959245304263703, 22.518873615560267, 25.35184036589849, 27.86907241582484, 30.09452231290066, 31.279132519962367, 31.42319896628056, 31.34047886165137, 31.01513754798293, 29.49962527749096, 27.416848987979705, 26.702811012859506, 26.761549035428136, 25.941086451086015, 24.137639746007082, 21.989981926119412, 19.82339126178258, 17.637342339374648, 15.317203628361016, 13.22935703513324, 11.987902868641605, 11.041818254131226, 9.369272721674168, 6.757041032110883, 4.168978378348772, 3.342019175109911, 3.924034123236837, 3.7993869351913023, 3.398609874619339, 2.6344642392674915, 2.208737926594062, 2.1958484988039295, 2.350473055233414, 1.7286260384491916], [-6.911774823333961, -9.189166577280433, -8.48239072021922, -6.010755095020188, -4.101448655851146, -3.0476590365744305, -3.6671281113856997, -4.485518579171492, -3.193710008119824, -2.1560032167800505, -3.107639070439321, -3.5367427447152755, -3.3779739322865034, -3.549569054020713, -3.4227006843281456, -3.0761711412486834, -3.3009115360654406, -3.638021251631293, -3.5695181641603186, -3.131520865459191, -3.233965986022651, -4.003136960250013, -4.49585285292539, -4.833483478495754, -5.975812669486849, -7.234673562544476, -6.984129807981538, -5.128295647796873, -4.288297818499789, -6.549258403495569, -8.432781909426868, -8.3365135529011, -8.666817656825442, -10.369661012462423, -11.022954466737593, -11.571377871571276, -13.006145635881332, -13.670937000910559, -14.265525463806394, -15.68496128938244, -17.13781686542378, -18.583498911519058, -19.073189471969414, -17.432954424592996, -15.914968797573055, -15.795789043823666, -15.407027138651564, -17.252039772225793, -22.007503850264587, -24.25647086229761, -22.913939066233315, -22.933973410669225, -24.840877857954283, -22.898708672883902, -18.74205714486301, -15.884121456166694, -13.40646132232781, -11.787111776962309, -11.390620900140705, -9.188613882657402, -4.17532673036961, 1.2697894413715964, 5.109262885955882, 7.428652713830848, 8.76883713586883, 9.011697083441176, 8.39323191172267, 7.858022419616741, 7.053593995443153, 4.641462131588517, 1.7667401375705154, 0.2585804752998886, 0.0697361753470851, 0.30005885403998356, 0.3547240222178729, -0.023265894869743065, -0.865112242164864, -2.3835826811688596, -4.765859808636186, -7.083307613379734, -8.230275925160587, -8.09968417802813, -7.621910762384674, -8.197950598041505, -8.794467362373162, -8.959111309460354, -8.427523952635251, -8.199473612556616, -7.332489076972176, -6.284065458171819, -5.075535848306625, -2.899189070124775]]} caption="Impulse Trace"
  out "FFT":cluster{"Time":dbl[], "Data":dbl[]}[](graph)=[{"Time"=[0.0, 2.4285714285714284, 4.857142857142857, 7.285714285714285, 9.714285714285714, 12.142857142857142, 14.57142857142857, 17.0, 19.428571428571427, 21.857142857142854, 24.285714285714285, 26.71428571428571, 29.14285714285714, 31.57142857142857, 34.0, 36.42857142857142, 38.857142857142854, 41.285714285714285, 43.71428571428571, 46.14285714285714, 48.57142857142857, 50.99999999999999, 53.42857142857142, 55.857142857142854, 58.28571428571428, 60.71428571428571, 63.14285714285714, 65.57142857142857, 68.0, 70.42857142857142, 72.85714285714285, 75.28571428571428, 77.71428571428571, 80.14285714285714, 82.57142857142857, 85.0, 87.42857142857142, 89.85714285714285, 92.28571428571428, 94.71428571428571, 97.14285714285714, 99.57142857142857, 101.99999999999999, 104.42857142857142, 106.85714285714285, 109.28571428571428], "Data"=[-1.3284468668364369, 0.0, -5.385537504125523, -15.435463954020964, -28.20242502234497, -36.188627418479825, -46.821100679629254, -59.82657648738342, -60.12789326773007, -67.74033305448545, -67.43236104125887, -73.91497262179129, -75.66943487606963, -80.89084510184429, -84.78362519917926, -80.28925937165945, -84.83816971087651, -90.841165394456, -92.1008770459143, -93.12969892427525, -93.1239884835098, -93.59722396846385, -94.23913883751817, -95.03481857879969, -95.9652928205479, -97.02957823967398, -98.25272314777915, -99.47408973138023, -100.67995536129459, -101.75168970423206, -102.45169383683884, -102.67175862402809, -102.42667398970796, -101.89963744051411, -101.23341265726822, -100.54134369942744, -99.89589291671743, -99.32464398191397, -98.80941732312183, -98.3845599371269, -98.02216433701514, -97.7428271179752, -97.51070308349362, -97.34863812476058, -97.23662707082708, -97.18682747785813]}, {"Time"=[0.0, 2.4285714285714284, 4.857142857142857, 7.285714285714285, 9.714285714285714, 12.142857142857142, 14.57142857142857, 17.0, 19.428571428571427, 21.857142857142854, 24.285714285714285, 26.71428571428571, 29.14285714285714, 31.57142857142857, 34.0, 36.42857142857142, 38.857142857142854, 41.285714285714285, 43.71428571428571, 46.14285714285714, 48.57142857142857, 50.99999999999999, 53.42857142857142, 55.857142857142854, 58.28571428571428, 60.71428571428571, 63.14285714285714, 65.57142857142857, 68.0, 70.42857142857142, 72.85714285714285, 75.28571428571428, 77.71428571428571, 80.14285714285714, 82.57142857142857, 85.0, 87.42857142857142, 89.85714285714285, 92.28571428571428, 94.71428571428571, 97.14285714285714, 99.57142857142857, 101.99999999999999, 104.42857142857142, 106.85714285714285, 109.28571428571428], "Data"=[-1.5496705664320274, 0.0, -4.860110798865151, -14.282620783168522, -30.77984931740528, -46.152219964000075, -51.95422232313002, -54.37045094711479, -54.82263024205827, -56.939406462948014, -62.58803271330898, -69.04431891242457, -71.35646170319595, -69.31080988780718, -69.19769930168579, -73.75025679111238, -75.43436652276954, -78.22382878323597, -77.30505871462772, -77.4337955930445, -90.41534302179403, -79.06350388121508, -89.74022697118966, -82.77935421878425, -85.42023054868396, -88.81641833576619, -84.9722965929378, -98.16214696949471, -86.03666163274603, -95.08964128350334, -87.96710398201944, -90.71299662271774, -90.85530527000452, -89.12997346851843, -93.43042420377094, -89.05470640032148, -93.14289027030972, -89.91021718566888, -91.4989677958443, -91.22960482915276, -90.40701070072812, -92.2785530886493, -90.14914566743471, -92.27569921170073, -90.58063748214397, -91.45162598511088]}, {"Time"=[0.0, 2.4285714285714284, 4.857142857142857, 7.285714285714285, 9.714285714285714, 12.142857142857142, 14.57142857142857, 17.0, 19.428571428571427, 21.857142857142854, 24.285714285714285, 26.71428571428571, 29.14285714285714, 31.57142857142857, 34.0, 36.42857142857142, 38.857142857142854, 41.285714285714285, 43.71428571428571, 46.14285714285714, 48.57142857142857, 50.99999999999999, 53.42857142857142, 55.857142857142854, 58.28571428571428, 60.71428571428571, 63.14285714285714, 65.57142857142857, 68.0, 70.42857142857142, 72.85714285714285, 75.28571428571428, 77.71428571428571, 80.14285714285714, 82.57142857142857, 85.0, 87.42857142857142, 89.85714285714285, 92.28571428571428, 94.71428571428571, 97.14285714285714, 99.57142857142857, 101.99999999999999, 104.42857142857142, 106.85714285714285, 109.28571428571428], "Data"=[-1.1664218302869287, 0.0, -5.7999172506159695, -16.126850733058582, -25.046922928293256, -32.57940677094908, -43.62012841003624, -51.40538416440961, -52.82432008730757, -59.501501613398204, -67.88449467820614, -78.99659078715906, -69.41618652327307, -75.15196131993586, -74.0700380184418, -87.48910401615639, -84.19029121292672, -76.94576506118878, -81.41337096617008, -80.48057330313488, -87.55783937149215, -86.20008175730692, -86.99251041734308, -91.02851016920489, -90.14406054396127, -93.18013132602485, -92.85697631201948, -98.18672656053016, -93.43503954782327, -103.11159327800384, -95.36797475598117, -96.72344771486891, -101.65587037623936, -95.16626707924362, -106.5303029807485, -96.74734219532563, -99.93694557726481, -101.22780556340504, -98.42705017903822, -106.91053176743132, -100.06534004060818, -104.41194040340267, -105.50714131162829, -102.99558788371621, -114.4491400824021, -105.55212320416854]}] caption="XY Graph"
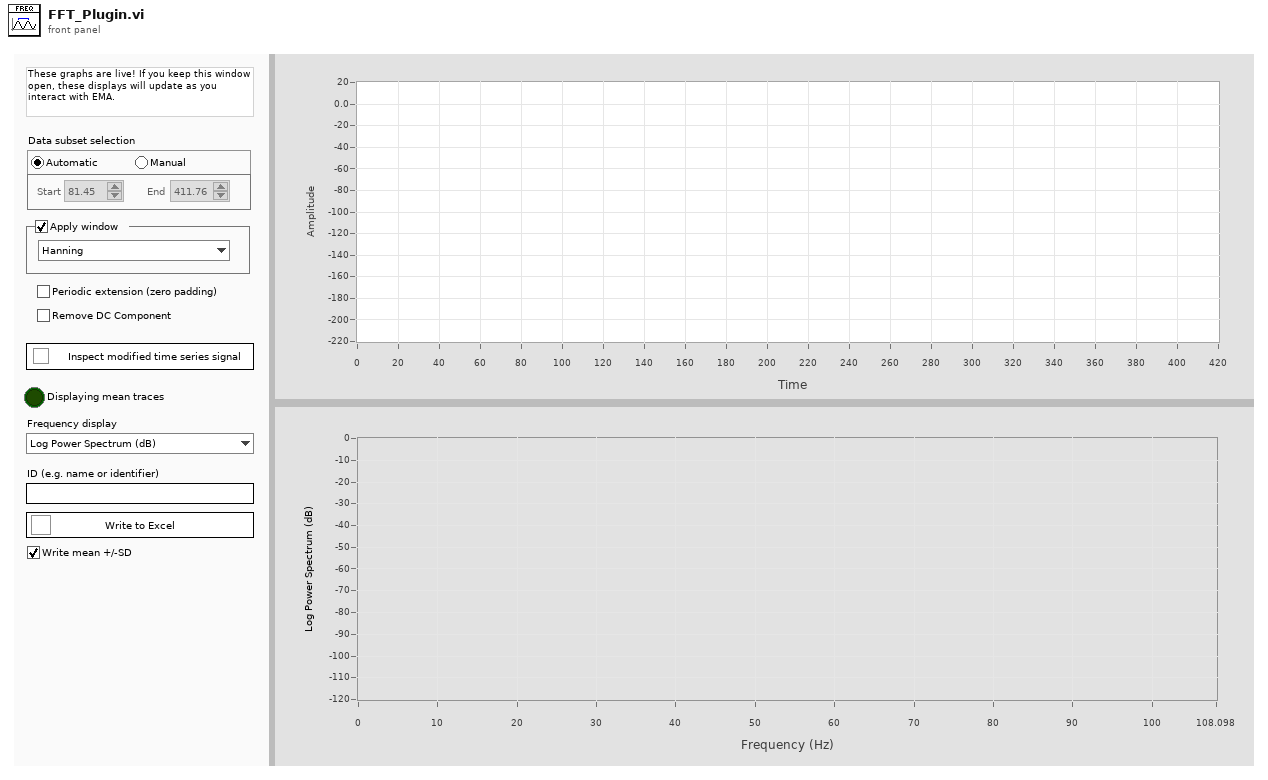
[diagram p1: front panel]
types:
  T1 = cluster{"Mean and STD":refnum<vi>, "Impulse dir":refnum<vi>, "Parameter Impuls Series":refnum<vi>, "Refresh":refnum<vi>}
  T2 = typedef "FFT_Plugin_states.ctl" = enum16{"Initialise", "Copy data", "Update cursors", "Perform FFT", "Launch inspection window", "Write to Excel", "Refresh", "Exit"}
  T3 = cluster{"Data header":string[], "Data":string[][], "Excel":refnum<class "Excel.lvclass">}
  T4 = typedef "LVMenuShortCut.ctl" = cluster{"Include Shift Key?":bool, "Include Ctrl Key?":bool, "Shortcut Key":string}
  T5 = cluster{"left":dbl, "top":dbl, "right":dbl, "bottom":dbl}
  T6 = cluster{"left":dbl, "top":dbl, "right":dbl, "bottom":dbl}[]
  T7 = cluster{"Horizontal":i32, "Vertical":i32, "Horizontal":i32, "Vertical":i32}[]
  T8 = enum32{"Invalid", "Standard", "Closed", "Hidden", "Minimized", "Maximized"}
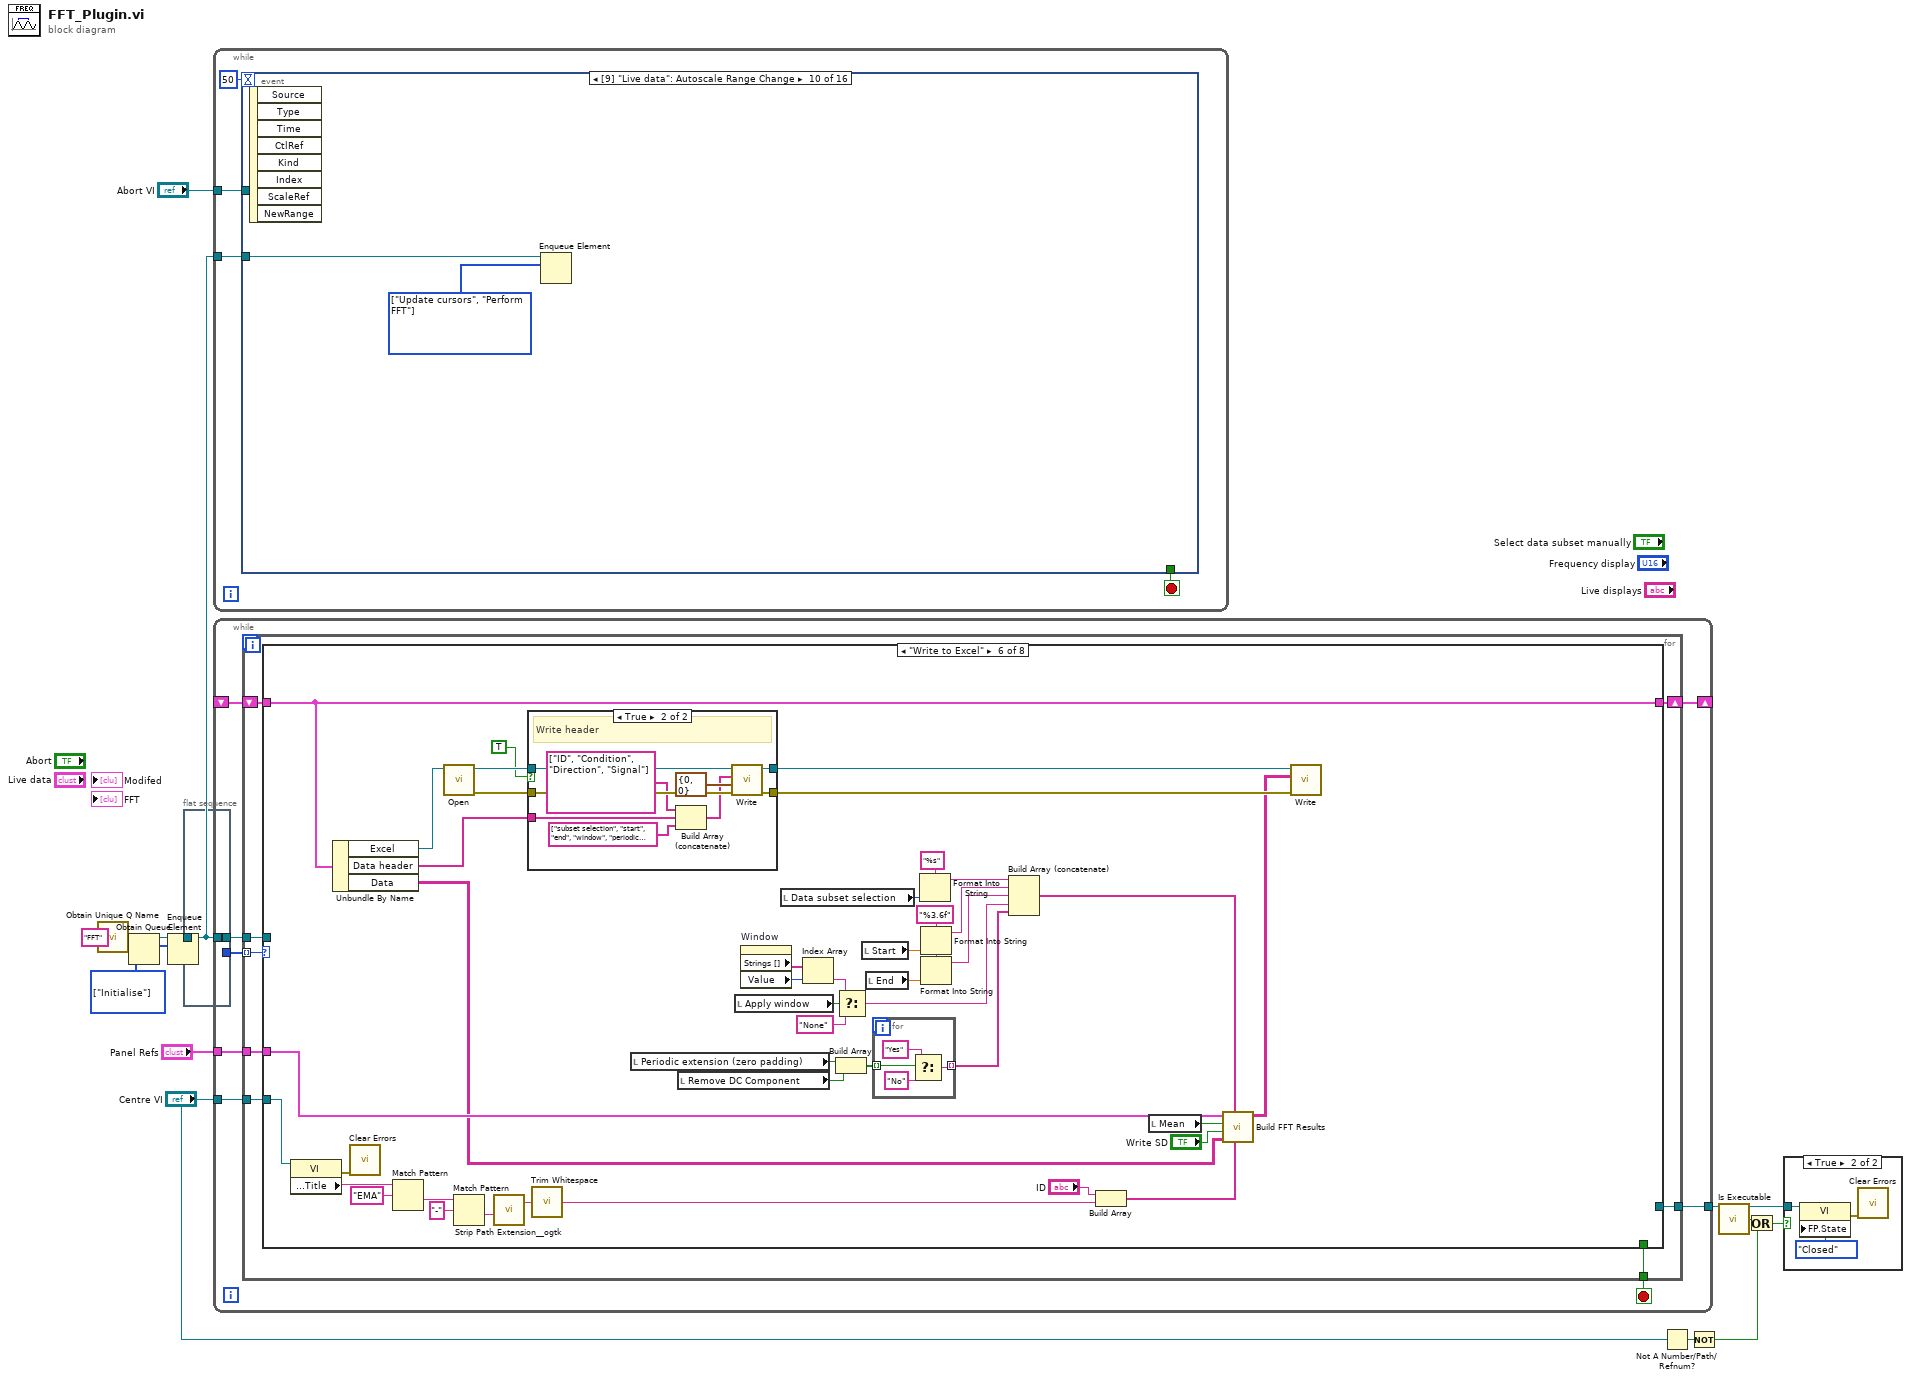
[diagram p0: block diagram]
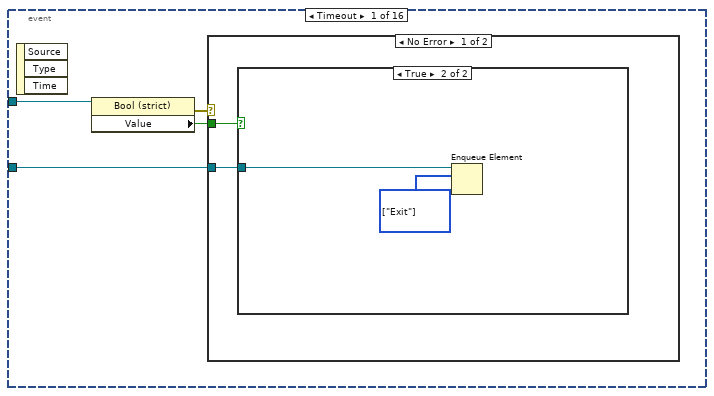
[diagram p2: hidden frame]
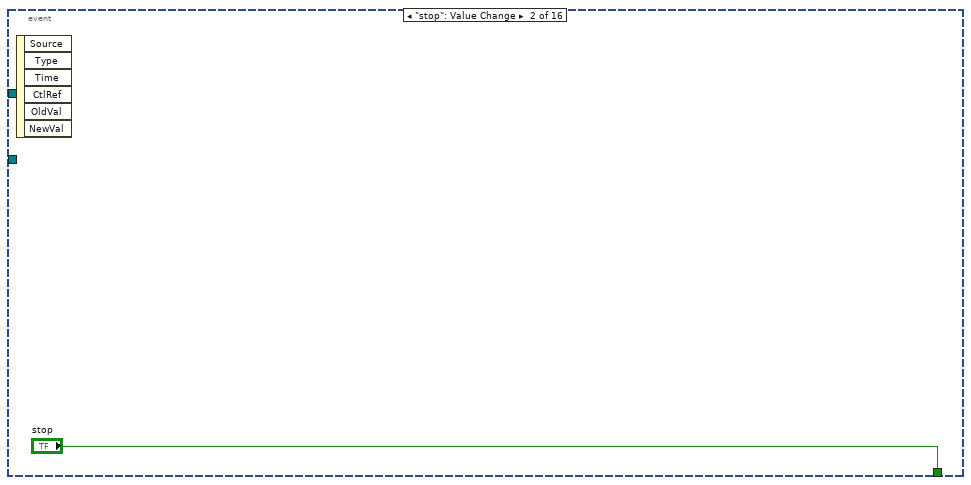
[diagram p5: hidden frame]
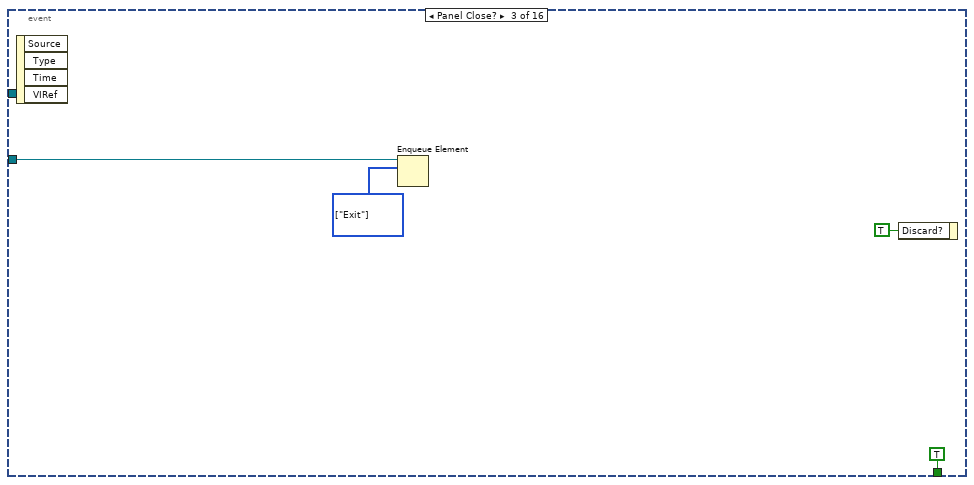
[diagram p6: hidden frame]
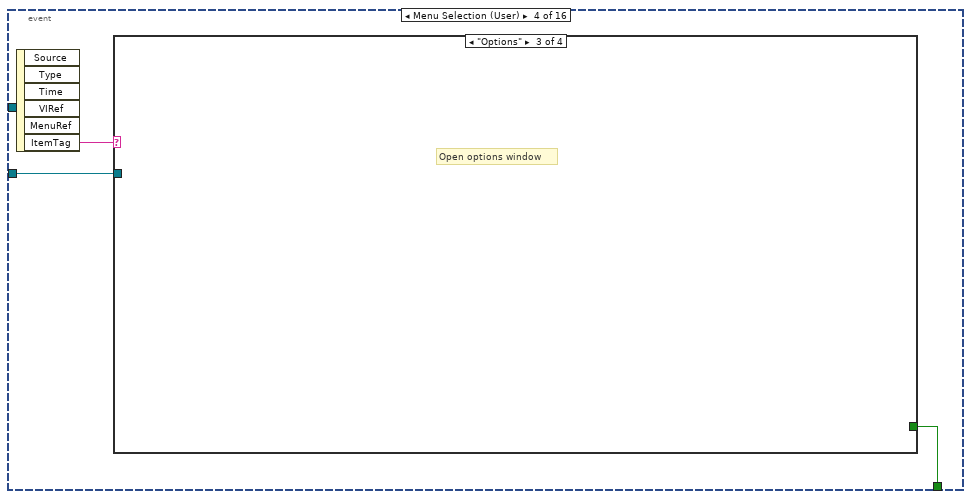
[diagram p7: hidden frame]
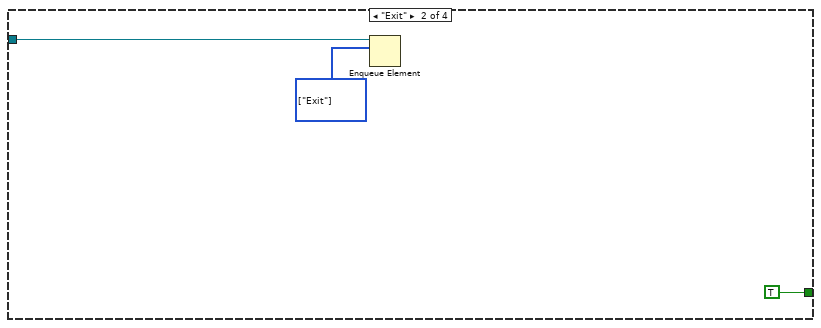
[diagram p9: hidden frame]
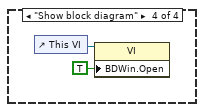
[diagram p10: hidden frame]
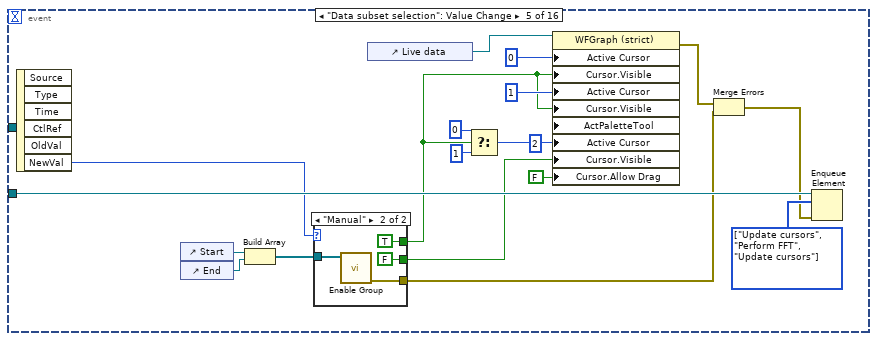
[diagram p11: hidden frame]
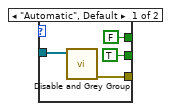
[diagram p12: hidden frame]
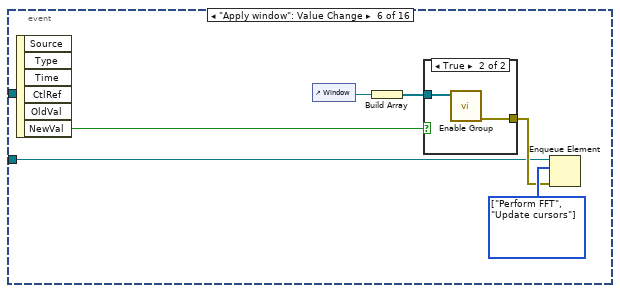
[diagram p13: hidden frame]
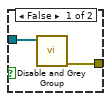
[diagram p14: hidden frame]
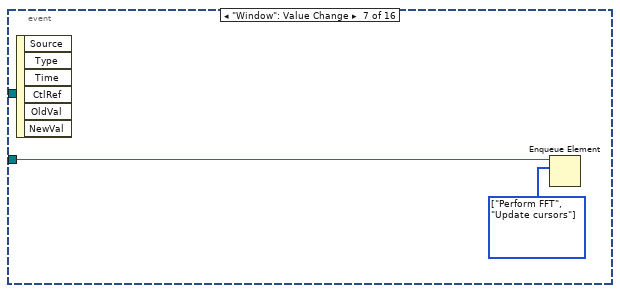
[diagram p15: hidden frame]
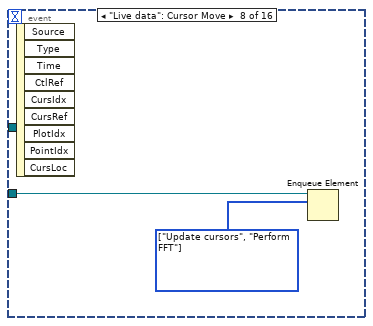
[diagram p16: hidden frame]
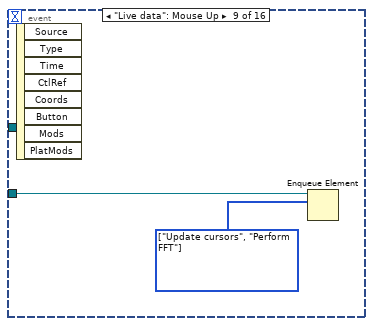
[diagram p17: hidden frame]
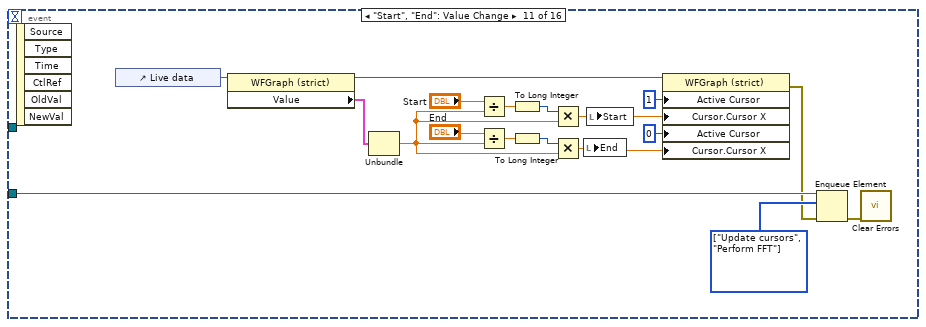
[diagram p18: hidden frame]
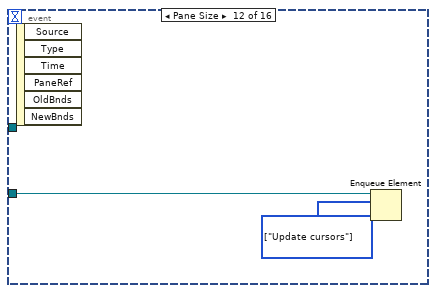
[diagram p19: hidden frame]
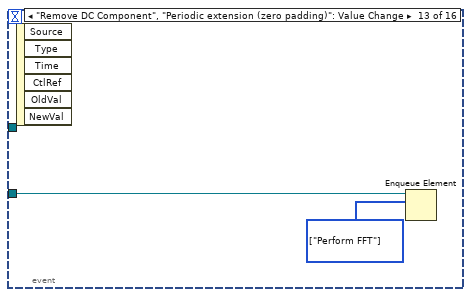
[diagram p20: hidden frame]
diagram:
  w10 = T2[] [enum."Initialise"] items=["Initialise", "Copy data", "Update cursors", "Perform FFT", "Launch inspection window", "Write to Excel", "Refresh", "Exit"]
  n1 = call <userlib>:"Obtain Unique Q Name.vi"("Queue"="FFT") -> ("Q Name"=w8:string)  [unwired: 4 in]
  n2 = Obtain Queue(name (unnamed)=w8, element data type=w10) -> (queue out=w9:refnum<queue>)  [unwired: 3 in, 2 out]
  n3 = Enqueue Element(queue=w9, element=w10) -> (queue out=w13:refnum<queue>)  [unwired: 2 in, 2 out]
  n4 = while {
    tunnel: w13 -> [w16]
    tunnel: "Abort VI" -> [w14]
    stop <- w17 stop-if-true
    n5 = event shown="[9] \"Live data\": Autoscale Range Change" {
      selector: _ -> [_ _ _ _ _ _ _ _ _ _ _ _ _ _ _ _]
      dyn-events: _ -> [_ _ _ _ _ _ _ _ _ _ _ _ _ _ _ _]
      timeout: 50 -> [_ _ _ _ _ _ _ _ _ _ _ _ _ _ _ _]
      tunnel: [_ "stop" TRUE w31 _ _ _ _ _ _ _ _ _ _ _ _] -> w17
      tunnel: w16 -> [w18 _ w29 w32 w52 w67 w76 w79 w81 w83 w91 w103 w105 w107 w109 w111]
      tunnel: w14 -> [w21 _ _ _ _ _ _ _ _ _ _ _ _ _ _ _]
      event Timeout {
        n6 = event-data() -> ()  [unwired: 1 in, 3 out]
        n7 = property class="Bool (strict)"(reference=w21) -> (error out=w19:errorcluster, "Value"=w20:bool)  [unwired: 1 in, 1 out]
        n8 = case shown="No Error" w19 {
          tunnel: w20 -> [w23 _]
          tunnel: w18 -> [w22 _]
          frame No Error {
            n9 = case shown="True" w23 {
              tunnel: w22 -> [_ w24]
              frame False {
              }
              frame True {
                w25 = T2[] [enum."Exit"] items=["Initialise", "Copy data", "Update cursors", "Perform FFT", "Launch inspection window", "Write to Excel", "Refresh", "Exit"]
                n10 = Enqueue Element(queue=w24, element=w25) -> ()  [unwired: 2 in, 3 out]
              }
            }
          }
          frame Error {
          }
        }
      }
      event "stop": Value Change {
        n11 = event-data() -> ()  [unwired: 1 in, 6 out]
      }
      event Panel Close? {
        w28 = T2[] [enum."Exit"] items=["Initialise", "Copy data", "Update cursors", "Perform FFT", "Launch inspection window", "Write to Excel", "Refresh", "Exit"]
        n12 = event-data() -> ()  [unwired: 1 in, 4 out]
        n13 = Enqueue Element(queue=w29, element=w28) -> ()  [unwired: 2 in, 3 out]
        n14 = event-data("Discard?"=TRUE) -> ()  [unwired: 1 in, 1 out]
      }
      event Menu Selection (User) {
        n15 = event-data() -> ("ItemTag"=w33:string)  [unwired: 1 in, 5 out]
        n16 = case shown="\"Options\"" w33 {
          tunnel: w32 -> [_ w36 _ _]
          tunnel: [_ TRUE _ _] -> w31
          frame Default {
          }
          frame "Exit" {
            w35 = T2[] [enum."Exit"] items=["Initialise", "Copy data", "Update cursors", "Perform FFT", "Launch inspection window", "Write to Excel", "Refresh", "Exit"]
            n17 = Enqueue Element(queue=w36, element=w35) -> ()  [unwired: 2 in, 3 out]
          }
          frame "Options" {
            # "Open options window"
          }
          frame "Show block diagram" {
            n18 = control-ref of="This VI"() -> (w38:refnum<vi>)
            n19 = property class="VI"(reference=w38, "BDWin.Open"=TRUE ("Block Diagram Window:Open")) -> ()  [unwired: 1 in, 2 out]
          }
        }
      }
      event "Data subset selection": Value Change {
        w51 = T2[] [enum."Update cursors", enum."Perform FFT", enum."Update cursors"] items=["Initialise", "Copy data", "Update cursors", "Perform FFT", "Launch inspection window", "Write to Excel", "Refresh", "Exit"]
        n20 = event-data() -> ("NewVal"=w43:enum32{"Automatic", "Manual"})  [unwired: 1 in, 5 out]
        n21 = control-ref of="Start"() -> (w54:refnum<vi>)
        n22 = control-ref of="End"() -> (w53:refnum<vi>)
        n23 = Build Array(w54, w53) -> (w55:refnum<vi>[])
        n24 = case shown="\"Manual\"" w43 {
          tunnel: w55 -> [w61 w65]
          tunnel: [w60 w64] -> w49
          tunnel: [FALSE TRUE] -> w42
          tunnel: [TRUE FALSE] -> w40
          frame "Automatic", Default {
            n25 = call <vilib>:"Disable and Grey Group.vi"("Group"=w61) -> ("error out"=w60:errorcluster)  [unwired: 9 in, 1 out]
          }
          frame "Manual" {
            n26 = call <vilib>:"Enable Group.vi"("Group"=w65) -> ("error out"=w64:errorcluster)  [unwired: 9 in, 1 out]
          }
        }
        n27 = control-ref of="Live data"() -> (w45:refnum<vi>)
        n28 = Select(t=0 ("Palette:Active Tool"), s=w42, f=1 ("Palette:Active Tool")) -> (s? t:f=w44:i32)
        n29 = property class="WFGraph (strict)"(reference=w45, "Active Cursor"=0, "Cursor.Visible"=w42, "Active Cursor"=1, "Cursor.Visible"=w42, "ActPaletteTool"=w44, "Active Cursor"=2, "Cursor.Visible"=w40, "Cursor.Allow Drag"=FALSE) -> (error out=w50:errorcluster)  [unwired: 1 in, 1 out]
        n30 = Merge Errors(w50, w49) -> (w48:errorcluster)
        n31 = Enqueue Element(queue=w52, element=w51, error in (no error)=w48) -> ()  [unwired: 1 in, 3 out]
      }
      event "Apply window": Value Change {
        w69 = T2[] [enum."Perform FFT", enum."Update cursors"] items=["Initialise", "Copy data", "Update cursors", "Perform FFT", "Launch inspection window", "Write to Excel", "Refresh", "Exit"]
        n32 = event-data() -> ("NewVal"=w71:bool)  [unwired: 1 in, 5 out]
        n33 = control-ref of="Window"() -> (w66:refnum<vi>)
        n34 = Build Array(w66) -> (w70:refnum<vi>[])
        n35 = case shown="True" w71 {
          tunnel: w70 -> [w73 w74]
          tunnel: [w72 w75] -> w68
          frame False {
            n36 = call <vilib>:"Disable and Grey Group.vi"("Group"=w73) -> ("error out"=w72:errorcluster)  [unwired: 9 in, 1 out]
          }
          frame True {
            n37 = call <vilib>:"Enable Group.vi"("Group"=w74) -> ("error out"=w75:errorcluster)  [unwired: 9 in, 1 out]
          }
        }
        n38 = Enqueue Element(queue=w67, element=w69, error in (no error)=w68) -> ()  [unwired: 1 in, 3 out]
      }
      event "Window": Value Change {
        w77 = T2[] [enum."Perform FFT", enum."Update cursors"] items=["Initialise", "Copy data", "Update cursors", "Perform FFT", "Launch inspection window", "Write to Excel", "Refresh", "Exit"]
        n39 = event-data() -> ()  [unwired: 1 in, 6 out]
        n40 = Enqueue Element(queue=w76, element=w77) -> ()  [unwired: 2 in, 3 out]
      }
      event "Live data": Cursor Move {
        w78 = T2[] [enum."Update cursors", enum."Perform FFT"] items=["Initialise", "Copy data", "Update cursors", "Perform FFT", "Launch inspection window", "Write to Excel", "Refresh", "Exit"]
        n41 = event-data() -> ()  [unwired: 1 in, 9 out]
        n42 = Enqueue Element(queue=w79, element=w78) -> ()  [unwired: 2 in, 3 out]
      }
      event "Live data": Mouse Up {
        w80 = T2[] [enum."Update cursors", enum."Perform FFT"] items=["Initialise", "Copy data", "Update cursors", "Perform FFT", "Launch inspection window", "Write to Excel", "Refresh", "Exit"]
        n43 = event-data() -> ()  [unwired: 1 in, 8 out]
        n44 = Enqueue Element(queue=w81, element=w80) -> ()  [unwired: 2 in, 3 out]
      }
      event "Live data": Autoscale Range Change {
        w82 = T2[] [enum."Update cursors", enum."Perform FFT"] items=["Initialise", "Copy data", "Update cursors", "Perform FFT", "Launch inspection window", "Write to Excel", "Refresh", "Exit"]
        n45 = event-data() -> ()  [unwired: 1 in, 8 out]
        n46 = Enqueue Element(queue=w83, element=w82) -> ()  [unwired: 2 in, 3 out]
      }
      event "Start", "End": Value Change {
        w92 = T2[] [enum."Update cursors", enum."Perform FFT"] items=["Initialise", "Copy data", "Update cursors", "Perform FFT", "Launch inspection window", "Write to Excel", "Refresh", "Exit"]
        n47 = event-data() -> ()  [unwired: 1 in, 6 out]
        n48 = control-ref of="Live data"() -> (w100:refnum<vi>)
        n49 = property class="WFGraph (strict)"(reference=w100) -> (reference out=w85:refnum<vi>, "Value"=w101:cluster{dbl, dbl, "Impulses":dbl[][]})  [unwired: 1 in, 1 out]
        n50 = Unbundle(w101) -> (w93:dbl)  [unwired: 2 out]
        n51 = Divide(x="Start", y=w93) -> (x/y=w99:dbl)
        n52 = Divide(x="End", y=w93) -> (x/y=w95:dbl)
        n53 = To Long Integer(number=w99) -> (32bit integer=w98:i32)
        n54 = To Long Integer(number=w95) -> (32bit integer=w96:i32)
        n55 = Multiply(x=w98, y=w93) -> (x*y=w89:dbl)
        n56 = Multiply(x=w96, y=w93) -> (x*y=w88:dbl)
        n57 = local write "End"(w88) -> ()
        n58 = local write "Start"(w89) -> ()
        n59 = property class="WFGraph (strict)"(reference=w85, "Active Cursor"=u32 1, "Cursor.Cursor X"=w89, "Active Cursor"=u32 0, "Cursor.Cursor X"=w88) -> (error out=w90:errorcluster)  [unwired: 1 in, 1 out]
        n60 = Enqueue Element(queue=w91, element=w92, error in (no error)=w90) -> (error out=w84:errorcluster)  [unwired: 1 in, 2 out]
        n61 = call <vilib>:"Clear Errors.vi"("error in (no error)"=w84) -> ()  [unwired: 5 in, 2 out]
      }
      event Pane Size {
        w102 = T2[] [enum."Update cursors"] items=["Initialise", "Copy data", "Update cursors", "Perform FFT", "Launch inspection window", "Write to Excel", "Refresh", "Exit"]
        n62 = event-data() -> ()  [unwired: 1 in, 6 out]
        n63 = Enqueue Element(queue=w103, element=w102) -> ()  [unwired: 2 in, 3 out]
      }
      event "Remove DC Component", "Periodic extension (zero padding)": Value Change {
        w104 = T2[] [enum."Perform FFT"] items=["Initialise", "Copy data", "Update cursors", "Perform FFT", "Launch inspection window", "Write to Excel", "Refresh", "Exit"]
        n64 = event-data() -> ()  [unwired: 1 in, 6 out]
        n65 = Enqueue Element(queue=w105, element=w104) -> ()  [unwired: 2 in, 3 out]
      }
      event "Inspect": Value Change {
        w106 = T2[] [enum."Launch inspection window"] items=["Initialise", "Copy data", "Update cursors", "Perform FFT", "Launch inspection window", "Write to Excel", "Refresh", "Exit"]
        n66 = event-data() -> ()  [unwired: 1 in, 6 out]
        n67 = Enqueue Element(queue=w107, element=w106) -> ()  [unwired: 2 in, 3 out]
      }
      event "Write to Excel": Value Change {
        w108 = T2[] [enum."Write to Excel"] items=["Initialise", "Copy data", "Update cursors", "Perform FFT", "Launch inspection window", "Write to Excel", "Refresh", "Exit"]
        n68 = event-data() -> ()  [unwired: 1 in, 6 out]
        n69 = Enqueue Element(queue=w109, element=w108) -> ()  [unwired: 2 in, 3 out]
      }
      event "Frequency display": Value Change {
        w110 = T2[] [enum."Perform FFT"] items=["Initialise", "Copy data", "Update cursors", "Perform FFT", "Launch inspection window", "Write to Excel", "Refresh", "Exit"]
        n70 = event-data() -> ()  [unwired: 1 in, 6 out]
        n71 = Enqueue Element(queue=w111, element=w110) -> ()  [unwired: 2 in, 3 out]
      }
    }
  }
  n72 = while {
    tunnel: w13 -> [w120]
    tunnel: [w116] -> w12
    shift-right: [w115] -> _
    shift-left: _ -> [w114]
    tunnel: "Centre VI" -> [w113]
    tunnel: "Panel Refs" -> [w112]
    stop <- w117 stop-if-true
    n73 = flat-sequence {
      tunnel: w120 -> [w127]
      tunnel: [w123] -> w118
      tunnel: [w126] -> w119
      frame #0 {
        w122 = T2[] [enum."Refresh"] items=["Initialise", "Copy data", "Update cursors", "Perform FFT", "Launch inspection window", "Write to Excel", "Refresh", "Exit"]
        n74 = Dequeue Element(queue=w127, timeout in ms (-1)=100) -> (queue out=w126:refnum<queue>, element=w121:T2[], timed out?=w124:bool)  [unwired: 1 in, 1 out]
        n75 = Select(t=w122, s=w124, f=w121) -> (s? t:f=w123:T2[])
      }
    }
    n76 = for {
      tunnel: w119 -> [w135]
      tunnel: w118 -> [w134] mode=indexing
      tunnel: [w133] -> w117
      tunnel: [w132] -> w116
      shift-right: [w131] -> w115
      shift-left: w114 -> [w130]
      tunnel: w113 -> [w129]
      tunnel: w112 -> [w128]
      n77 = case shown="\"Write to Excel\"" w134 {
        tunnel: w135 -> [w138 _ _ _ _ _ w448 _]
        tunnel: [_ _ _ _ _ _ _ TRUE] -> w133
        tunnel: [_ _ _ _ _ _ _ w457] -> w132
        tunnel: [w137 w214 w248 w264 w378 w421 w449 w455] -> w131
        tunnel: w130 -> [_ w214 w248 w265 w378 w421 w449 w455]
        tunnel: w129 -> [w136 w206 _ _ _ w413 _ _]
        tunnel: w128 -> [_ w194 _ _ _ w406 w443 _]
        frame "Initialise", Default {
          n78 = stacked-sequence {
            tunnel: w138 -> [_ _ _ w178]
            tunnel: [_ w146 _ _] -> w137
            tunnel: w136 -> [w139 _ _ _]
            frame #0 {
              # "Initialise"
              n79 = call <userlib>:"Centre window relative to caller.vi"("Enable (T)"=TRUE, "VI reference"=w139) -> ()  [unwired: 3 in, 1 out]
              n80 = local write "stop"(FALSE ("stop")) -> ()
              n81 = local write "Abort"(FALSE ("stop")) -> ()
              n82 = control-ref of="Live data"() -> (w142:refnum<vi>)
              n83 = property class="WFGraph (strict)"(reference=w142, "PlotImages.Front"=picture data[5B] ("Plot Images:Front")) -> ()  [unwired: 1 in, 2 out]
            }
            frame #1 {
              # "Build Program Cluster"
              n84 = call <userlib>:"Create.vi"() -> ("Excel out"=w145:refnum<class "Excel.lvclass">)  [unwired: 10 in, 1 out]
              n85 = Bundle By Name(cluster=T3 {"Data header"=["-3dB freq [0]", "-3dB freq [1]", "-6dB freq [0]", "-6dB freq [1]", "-9dB freq [0]", "-9dB freq [1]", "peak freq [0]", "peak power [0]", "peak freq [1]", "peak power [1]", "peak freq [2]", "peak power [2]"], "Data"=[], "Excel"=refnum} ("Program Cluster"), "Excel"=w145) -> (w146:T3)
            }
            frame #2 {
              # "Setup Menu"
              n86 = Current VI's Menubar() -> (w161:refnum<k9>)
              n87 = Delete Menu Items(9:w161) -> (3:w160:refnum<k9>)  [unwired: 3 in, 1 out]
              n88 = Insert Menu Items(7:string[] ["File", "Tools"] ("item tags"), 9:w160) -> (3:w159:refnum<k9>)  [unwired: 4 in, 2 out]
              n89 = Insert Menu Items(5:"File" ("menu tag"), 7:string[] ["Exit"] ("item tags"), 9:w159) -> (1:w152:string[], 3:w155:refnum<k9>)  [unwired: 3 in, 1 out]
              n90 = Insert Menu Items(5:"Tools" ("menu tag"), 7:string[] ["Options"] ("item tags"), 9:w155) -> (3:w150:refnum<k9>)  [unwired: 3 in, 2 out]
              n91 = for {
                tunnel: w150 -> [w176]
                tunnel: w152 -> [w175] mode=indexing
                tunnel: T4[] [{"Include Shift Key?"=FALSE, "Include Ctrl Key?"=TRUE, "Shortcut Key"="x"}] -> [w174] mode=indexing
                tunnel: [w173] -> w149
                n92 = Set Menu Item Info(4:w174, 7:w175, 11:w176) -> (3:w173:refnum<k9>)  [unwired: 4 in, 1 out]
              }
              n93 = call <userlib>:"Is Executable.vi"() -> ("exe?"=w148:bool)  [unwired: 5 in]
              n94 = case shown="False" w148 {
                tunnel: w149 -> [w165 _]
                frame False {
                  # "Development-only menu"
                  n95 = Insert Menu Items(7:string[] ["Development"] ("item tags"), 9:w165) -> (3:w164:refnum<k9>)  [unwired: 4 in, 2 out]
                  n96 = Insert Menu Items(5:"Development" ("menu tag"), 7:string[] ["Show block diagram"] ("item tags"), 9:w164) -> (1:w166:string[], 3:w168:refnum<k9>)  [unwired: 3 in, 1 out]
                  n97 = for {
                    tunnel: w168 -> [w172]
                    tunnel: T4[] [{"Include Shift Key?"=FALSE, "Include Ctrl Key?"=TRUE, "Shortcut Key"="e"}] -> [w171] mode=indexing
                    tunnel: w166 -> [w170] mode=indexing
                    n98 = Set Menu Item Info(4:w171, 7:w170, 11:w172) -> ()  [unwired: 4 in, 2 out]
                  }
                }
                frame True {
                }
              }
            }
            frame #3 {
              w177 = T2[] [enum."Copy data", enum."Update cursors", enum."Perform FFT", enum."Update cursors"] items=["Initialise", "Copy data", "Update cursors", "Perform FFT", "Launch inspection window", "Write to Excel", "Refresh", "Exit"]
              # "Enqueue Initial States"
              n99 = Enqueue Element(queue=w178, element=w177) -> ()  [unwired: 2 in, 3 out]
            }
          }
        }
        frame "Copy data" {
          # "The invisible 4th cursor is always at the end of the file"
          n100 = property class="VI"(reference=w206) -> (error out=w207:errorcluster, "Front Panel.Title"=w213:string)  [unwired: 1 in, 1 out]
          n101 = call <vilib>:"Clear Errors.vi"("error in (no error)"=w207) -> ()  [unwired: 5 in, 2 out]
          n102 = Unbundle By Name(w194) -> ("Mean and STD"=w195:refnum<vi>)
          n103 = Match Pattern(string=w213, regular expression="EMA") -> (after substring=w211:string)  [unwired: 1 in, 3 out]
          n104 = Match Pattern(string=w211, regular expression="-") -> (after substring=w209:string)  [unwired: 1 in, 3 out]
          n105 = call-poly <userlib>:"Strip Path Extension__ogtk.vi"("path"=w209) -> ("root"=w208:string)  [unwired: 1 out]
          n106 = property class="Bool"(reference=w195) -> (error out=w198:errorcluster, "Value"=w196:variant)  [unwired: 1 in, 1 out]
          n107 = call <vilib>:"Trim Whitespace.vi"("string"=w208) -> ("trimmed string"=w203:string)  [unwired: 1 in]
          n108 = Empty String/Path?(string/path=w203) -> (empty?=w202:bool)
          n109 = Concatenate Strings("Fourier Transform :: " ("string"), w203) -> (w200:string)
          n110 = Variant To Data(error in=w198, type=TRUE, Variant=w196) -> (data=w193:bool, error out=w192:errorcluster)
          "Mean" <- w193
          n111 = Select(t="Fourier Transform" ("string"), s=w202, f=w200) -> (s? t:f=w199:string)
          n112 = control-ref of="This VI"() -> (w205:refnum<vi>)
          n113 = property class="VI"(reference=w205, "Front Panel.Title"=w199) -> ()  [unwired: 1 in, 2 out]
          n114 = property on="Write SD" class="Bool (strict)"(error in=w192, "Visible"=w193) -> (error out=w191:errorcluster)  [unwired: 1 in, 1 out]
          n115 = control-ref of="Live data"() -> (w189:refnum<vi>)
          n116 = call <vilib>:"Clear Errors.vi"("error in (no error)"=w191) -> ()  [unwired: 5 in, 2 out]
          n117 = property class="WFGraph (strict)"(reference="Data reference") -> (reference out=w190:refnum<vi>, error out=w186:errorcluster, "Value"=w187:cluster{dbl, dbl, "Impulses":dbl[][]})  [unwired: 1 in]
          n118 = property class="WFGraph (strict)"(reference=w189, error in=w186, "Value"=w187) -> (reference out=w188:refnum<vi>, error out=w185:errorcluster)
          n119 = call "Copy Graph Attributes.vi"("error in (no error)"=w185, "Copy to"=w188, "Copy from"=w190) -> ("error out"=w183:errorcluster)  [unwired: 8 in]
          n120 = call <vilib>:"Clear Errors.vi"("error in (no error)"=w183) -> ("error out"=w181:errorcluster)  [unwired: 5 in, 1 out]
          n121 = property on="Live data" class="WFGraph (strict)"(error in=w181, "Active Cursor"=u32 3, "Cursor.Cursor X"=10000000.0 ("Cursor.Cursor Position:Cursor X")) -> ("Cursor.Cursor X"=w179:dbl)  [unwired: 1 in, 2 out]
          n122 = local write "End"(w179) -> ()
        }
        frame "Update cursors" {
          w230 = T5 {"left"=0.0, "top"=0.0, "right"=200.0, "bottom"=200.0} ("rect")
          # "Draw greyed-out region to indicate cursor location\n(region of file that has been cut)"
          n123 = local read "Data subset selection"() -> (w217:enum32{"Automatic", "Manual"})
          n124 = case shown="\"Automatic\", Default" w217 {
            tunnel: [2 1] -> w216
            tunnel: [3 0] -> w215
            frame "Automatic", Default {
            }
            frame "Manual" {
            }
          }
          n125 = control-ref of="This VI"() -> (w239:refnum<vi>)
          n126 = property class="VI"(reference=w239) -> ("Panel"=w238:refnum<vi>)  [unwired: 1 in, 2 out]
          n127 = control-ref of="Live data"() -> (w231:refnum<vi>)
          n128 = property class="Pnl"(reference=w238, "DeferPanUpdts"=TRUE ("Defer Panel Updates")) -> (reference out=w234:refnum<vi>, error out=w236:errorcluster)  [unwired: 1 in]
          n129 = property class="WFGraph (strict)"(reference=w231, error in=w236, "Active Cursor"=w216, "Active Cursor"=w215, "ActYScl"=0) -> (reference out=w245:refnum<vi>, error out=w244:errorcluster, "Cursor.Cursor X"=w247:dbl, "Cursor.Cursor X"=w246:dbl, "XScale.Maximum"=w241:dbl, "YScale.Maximum"=w243:dbl, "YScale.Minimum"=w242:dbl)
          n130 = Build Array(w247, w246) -> (w229:dbl[])
          n131 = Array Max & Min(array=w229) -> (max value=w224:dbl, min value=w228:dbl)  [unwired: 2 out]
          n132 = Bundle By Name(cluster=w230, "left"=0.0, "top"=w243, "right"=w228, "bottom"=w242) -> (w227:T5)
          n133 = Bundle By Name(cluster=w230, "left"=w224, "top"=w243, "right"=w241, "bottom"=w242) -> (w226:T5)
          n134 = Build Array(w227, w226) -> (w220:T6)
          n135 = call "Overlay XY Position to Coords.vi"("XY"=w220, "Graph"=w245) -> ("Coords"=w219:T7, "Graph out"=w221:refnum<vi>)  [unwired: 8 in]
          n136 = call "Empty Picture"() -> ("empty picture"=w218:picture)
          n137 = for {
            tunnel: w219 -> [w256] mode=indexing
            tunnel: u32 13027014 ("color(black)") -> [w255]
            shift-right: [w254] -> w223
            shift-left: w218 -> [w253]
            n138 = call <vilib>:"Draw Grayed Out Rect.vi"("color(black)"=w255, "rect"=w256, "picture"=w253) -> ("new picture"=w254:picture)  [unwired: 2 in]
          }
          n139 = property class="WFGraph"(reference=w221, error in=w244, "Active Cursor"=w216, "Cursor.Cursor X"=w247, "Active Cursor"=w215, "Cursor.Cursor X"=w246, "PlotImages.Front"=w223) -> (error out=w232:errorcluster)  [unwired: 1 out]
          n140 = property class="Pnl"(reference=w234, error in=w232, "DeferPanUpdts"=FALSE ("Defer Panel Updates")) -> (error out=w233:errorcluster)  [unwired: 1 out]
          n141 = call <vilib>:"Clear Errors.vi"("error in (no error)"=w233) -> ()  [unwired: 5 in, 2 out]
          n142 = local write "Start"(w247) -> ()
          n143 = local write "End"(w246) -> ()
        }
        frame "Perform FFT" {
          n144 = control-ref of="Live data"() -> (w257:refnum<vi>)
          n145 = call "Select visible data.vi"("Data ref"=w257) -> ("Cursors"=w261:dbl[], "dt"=w260:dbl, "Visible Data"=w259:dbl[][])  [unwired: 8 in]
          n146 = for {
            tunnel: w259 -> [w318] mode=indexing
            tunnel: w260 -> [w319]
            tunnel: w261 -> [w317]
            tunnel: "Apply window" -> [w307]
            tunnel: "Remove DC Component" -> [w316]
            tunnel: "Periodic extension (zero padding)" -> [w315]
            tunnel: [w314] -> w270 mode=indexing
            tunnel: [w306] -> w278 mode=indexing
            tunnel: [w300] -> w271 mode=indexing
            tunnel: [w295] -> w266 mode=indexing
            tunnel: [w291] -> w263
            tunnel: [w290] -> w262 mode=indexing
            tunnel: "Data subset selection" -> [w289]
            tunnel: w257 -> [w288]
            i -> [w287]
            # "convert ms to seconds"
            n147 = case shown="\"Automatic\", Default" w289 {
              tunnel: [w340 w349] -> w311
              tunnel: w318 -> [w344 w357]
              tunnel: w319 -> [w337 w355]
              tunnel: w317 -> [_ w354]
              tunnel: w288 -> [w339 _]
              tunnel: w287 -> [w336 _]
              frame "Automatic", Default {
                n148 = call "Onset detection.vi"("dt"=w337, "Data"=w344) -> ("Cursor X"=w338:dbl, "Onset index"=w343:i32, "Data out"=w341:dbl[])  [unwired: 6 in, 1 out]
                n149 = case shown="0" w336 {
                  tunnel: w339 -> [_ w347]
                  tunnel: w338 -> [_ w346]
                  frame 1, Default {
                  }
                  frame 0 {
                    n150 = property class="WFGraph (strict)"(reference=w347, "Active Cursor"=u32 2, "Cursor.Cursor X"=w346) -> ()  [unwired: 1 in, 2 out]
                  }
                }
                n151 = Array Size(array=w341) -> (size(s)=w342:i32)
                n152 = Delete From Array(array=w341, length=w342, index=w343) -> (deleted portion=w340:dbl[])  [unwired: 1 out]
              }
              frame "Manual" {
                n153 = Divide(x=w354, y=w355) -> (x/y=w356:dbl[])
                n154 = To Long Integer(number=w356) -> (32bit integer=w353:i32[])
                n155 = Array Max & Min(array=w353) -> (max value=w352:i32, min value=w351:i32)  [unwired: 2 out]
                n156 = Subtract(x=w352, y=w351) -> (x-y=w350:i32)
                n157 = Increment(x=w350) -> (x+1=w348:i32)
                n158 = Delete From Array(array=w357, length=w348, index=w351) -> (deleted portion=w349:dbl[])  [unwired: 1 out]
              }
            }
            n159 = case shown="True" w316 {
              tunnel: w311 -> [w332 w334]
              tunnel: [w332 w333] -> w310
              frame False {
              }
              frame True {
                n160 = call-poly <vilib>:"Mean.vi"("X"=w334) -> ("mean"=w335:dbl)  [unwired: 1 out]
                n161 = Subtract(x=w334, y=w335) -> (x-y=w333:dbl[])
              }
            }
            n162 = case shown="True" w307 {
              tunnel: w310 -> [w323 w326]
              tunnel: [w323 w325] -> w309
              tunnel: "Window" -> [_ w324]
              frame False {
              }
              frame True {
                n163 = call-poly <vilib>:"Scaled Time Domain Window.vi"("window"=w324, "X"=w326) -> ("Windowed X"=w325:dbl[])  [unwired: 7 in, 2 out]
              }
            }
            n164 = case shown="True" w315 {
              tunnel: [w327 w331] -> w294
              tunnel: w309 -> [w327 w329]
              frame False {
              }
              frame True {
                w328 = 10000 ("post")
                n165 = call <userlib>:"Pad Array.vi"("Padding type"=enum16{"Duplicate ends", "Zeroes"}."Zeroes", "post"=w328, "pre"=w328, "Array"=w329) -> ("Padded array"=w331:dbl[])  [unwired: 4 in, 3 out]
              }
            }
            n166 = Divide(x=w319, y=1000.0) -> (x/y=w313:dbl)
            n167 = call <vilib>:"Auto Power Spectrum.vi"("dt"=w313, "Signal (V)"=w294) -> ("df"=w292:dbl, "Power Spectrum (V^2 rms)"=w293:dbl[])
            n168 = Logarithm Base 10(1:w293) -> (0:w304:dbl[])
            n169 = Add Array Elements(numeric array=w293) -> (sum=w297:dbl)
            n170 = Multiply(x=w304, y=10.0) -> (x*y=w302:dbl[])
            n171 = Divide(x=w293, y=w297) -> (x/y=w296:dbl[])
            n172 = for {
              tunnel: w296 -> [w321] mode=indexing
              shift-right: [w320] -> _
              shift-left: 0.0 -> [w322]
              tunnel: [w320] -> w299 mode=indexing
              n173 = Add(x=w321, y=w322) -> (x+y=w320:dbl)
            }
            n174 = Array Max & Min(array=w302) -> (max value=w303:dbl)  [unwired: 3 out]
            n175 = Subtract(x=w302, y=w303) -> (x-y=w301:dbl[])
            n176 = call "FFT_Summary_to_String.vi"("df"=w292, "Power Spectrum (V^2 rms)"=w293) -> ("Data"=w290:string[], "Header"=w291:string[])  [unwired: 8 in]
            n177 = call <userlib>:"Build XY Display.vi"("dt"=w319, "Data"=w294) -> ("Data"=w306:cluster{"Time":dbl[], "Data":dbl[]})  [unwired: 6 in, 3 out]
            n178 = call <userlib>:"Build XY Display.vi"("dt"=w292, "Data"=w293) -> ("Data"=w314:cluster{"Time":dbl[], "Data":dbl[]})  [unwired: 6 in, 3 out]
            n179 = call <userlib>:"Build XY Display.vi"("dt"=w292, "Data"=w301) -> ("Data"=w300:cluster{"Time":dbl[], "Data":dbl[]})  [unwired: 6 in, 3 out]
            n180 = call <userlib>:"Build XY Display.vi"("dt"=w292, "Data"=w299) -> ("Data"=w295:cluster{"Time":dbl[], "Data":dbl[]})  [unwired: 6 in, 3 out]
          }
          n181 = Build Array(w271, w270, w266) -> (w269:cluster{"Time":dbl[], "Data":dbl[]}[][])
          n182 = Bundle By Name(cluster=w265, "Data header"=w263, "Data"=w262) -> (w264:T3)
          n183 = control-ref of="Modifed"() -> (w279:refnum<vi>)
          n184 = control-ref of="FFT"() -> (w282:refnum<vi>)
          n185 = property on="Frequency display" class="Ring (strict)"() -> ("Strings []"=w273:string[], "Value"=w268:u16)  [unwired: 2 in, 2 out]
          n186 = property on="Property Node" class="XYGraph (strict)"(reference=w279, "Value"=w278) -> (reference out=w276:refnum<vi>, error out=w277:errorcluster)  [unwired: 1 in]
          n187 = Index Array(array=w269, index (row)=w268) -> (element=w267:cluster{"Time":dbl[], "Data":dbl[]}[])  [unwired: 1 in]
          n188 = Index Array(array=w273, index=w268) -> (element=w272:string)
          n189 = property on="Property Node" class="XYGraph (strict)"(reference=w282, "Value"=w267, "YScale.NameLbl.Text"=w272) -> (reference out=w281:refnum<vi>, error out=w283:errorcluster)  [unwired: 1 in]
          n190 = control-ref of="Live data"() -> (w274:refnum<vi>)
          n191 = call "Copy Graph Attributes.vi"("error in (no error)"=w277, "Copy to"=w276, "Copy from"=w274) -> ("error out"=w275:errorcluster)  [unwired: 8 in]
          n192 = call "Copy Graph Attributes.vi"("error in (no error)"=w283, "Copy to"=w281, "Copy from"=w274) -> ("error out"=w280:errorcluster)  [unwired: 8 in]
          n193 = call <vilib>:"Clear Errors.vi"("error in (no error)"=w275) -> ()  [unwired: 5 in, 2 out]
          n194 = call <vilib>:"Clear Errors.vi"("error in (no error)"=w280) -> ()  [unwired: 5 in, 2 out]
        }
        frame "Launch inspection window" {
          # "Allow time for a possibly running instance of this VI to close"
          n195 = control-ref of="Abort"() -> (w362:refnum<vi>)
          n196 = property class="Bool (strict)"(reference=w362, "Value"=TRUE) -> (reference out=w370:refnum<vi>, error out=w373:errorcluster)  [unwired: 1 in]
          n197 = call <userlib>:"inline delay.vi"("milliseconds to wait"=u32 100, "error in"=w373) -> ("error out"=w369:errorcluster)  [unwired: 7 in, 1 out]
          n198 = property class="Bool (strict)"(reference=w370, error in=w369, "Value"=FALSE) -> (error out=w368:errorcluster)  [unwired: 1 out]
          n199 = call <userlib>:"Current VIs Parent Directory__ogtk.vi"() -> ("Parent Directory (+ Relative)"=w358:path)  [unwired: 5 in]
          n200 = Build Path(base path=w358, name or relative path="subvi") -> (appended path=w365:path)
          n201 = Build Path(base path=w365, name or relative path="Time_series_exam.vi") -> (appended path=w363:path)
          n202 = Open VI Reference(type specifier VI Refnum (for type only)=refnum<vi> refnum, vi path=w363, options=128, error in (no error)=w368) -> (vi reference=w376:refnum<vi>, error out=w371:errorcluster)  [unwired: 2 in]
          n203 = control-ref of="Modifed"() -> (w359:refnum<vi>)
          n204 = control-ref of="Abort"() -> (w360:refnum<vi>)
          n205 = control-ref of="This VI"() -> (w361:refnum<vi>)
          n206 = call-by-ref "Start Asynchronous Call"(reference=w376, error in=w371, "Plot reference"=w359, "Abort"=w360, "Centre VI"=w361) -> ()  [unwired: 8 in, 3 out]
        }
        frame "Write to Excel" {
          w397 = "%3.6f" ("format string")
          n207 = property class="VI"(reference=w413) -> (error out=w410:errorcluster, "Front Panel.Title"=w419:string)  [unwired: 1 in, 1 out]
          n208 = Unbundle By Name(w421) -> ("Excel"=w420:refnum<class "Excel.lvclass">, "Data header"=w409:string[], "Data"=w403:string[][])
          n209 = call <vilib>:"Clear Errors.vi"("error in (no error)"=w410) -> ()  [unwired: 5 in, 2 out]
          n210 = Match Pattern(string=w419, regular expression="EMA") -> (after substring=w417:string)  [unwired: 1 in, 3 out]
          n211 = call <userlib>:"Open.vi"("Excel in"=w420) -> ("error out"=w411:errorcluster, "Excel out"=w412:refnum<class "Excel.lvclass">)  [unwired: 9 in]
          n212 = Match Pattern(string=w417, regular expression="-") -> (after substring=w415:string)  [unwired: 1 in, 3 out]
          n213 = call-poly <userlib>:"Strip Path Extension__ogtk.vi"("path"=w415) -> ("root"=w414:string)  [unwired: 1 out]
          n214 = case shown="True" TRUE {
            tunnel: w411 -> [w426 w436]
            tunnel: w412 -> [w427 w435]
            tunnel: w409 -> [_ w432]
            tunnel: [w427 w430] -> w408
            tunnel: [w426 w429] -> w407
            frame False {
              # "Header exists"
            }
            frame True {
              # "Write header"
              n215 = Build Array (concatenate)(string[] ["ID", "Condition", "Direction", "Signal"], w432, string[] ["subset selection", "start", "end", "window", "periodic extension", "DC offset removed"]) -> (w431:string[])
              n216 = call <userlib>:"Write.vi"("error in (no error)"=w436, "Cell (Append to next row)"=cluster{"Row":i32, "Col":i32} {"Row"=0, "Col"=0}, "Data"=w431, "Excel in"=w435) -> ("error out"=w429:errorcluster, "Excel out"=w430:refnum<class "Excel.lvclass">)  [unwired: 6 in]
            }
          }
          n217 = call <vilib>:"Trim Whitespace.vi"("string"=w414) -> ("trimmed string"=w381:string)  [unwired: 1 in]
          n218 = local read "Periodic extension (zero padding)"() -> (w386:bool)
          n219 = local read "Remove DC Component"() -> (w385:bool)
          n220 = local read "Apply window"() -> (w390:bool)
          n221 = property on="Window" class="Ring (strict)"() -> ("Strings []"=w392:string[], "Value"=w391:u16)  [unwired: 2 in, 2 out]
          n222 = local read "Data subset selection"() -> (w396:enum32{"Automatic", "Manual"})
          n223 = Index Array(array=w392, index=w391) -> (element=w389:string)
          n224 = Build Array(w386, w385) -> (w384:bool[])
          n225 = Select(t=w389, s=w390, f="None") -> (s? t:f=w387:string)
          n226 = local read "Start"() -> (w401:dbl)
          n227 = local read "End"() -> (w400:dbl)
          n228 = for {
            tunnel: w384 -> [w425] mode=indexing
            tunnel: [w422] -> w383 mode=indexing
            n229 = Select(t="Yes", s=w425, f="No") -> (s? t:f=w422:string)
          }
          n230 = Format Into String(format string="%s", w396) -> (resulting string=w394:string)  [unwired: 2 in, 1 out]
          n231 = Format Into String(format string=w397, w401) -> (resulting string=w399:string)  [unwired: 2 in, 1 out]
          n232 = Format Into String(format string=w397, w400) -> (resulting string=w398:string)  [unwired: 2 in, 1 out]
          n233 = Build Array (concatenate)(w394, w399, w398, w387, w383) -> (w393:string[])
          n234 = Build Array("ID", w381) -> (w380:string[])
          n235 = local read "Mean"() -> (w404:bool)
          n236 = call "Build FFT Results.vi"("ID/Condition"=w380, "data info"=w393, "Freq data"=w403, "Write SD"="Write SD", "Mean"=w404, "Panel Refs"=w406) -> ("FFT Results"=w402:string[][])  [unwired: 5 in]
          n237 = call <userlib>:"Write.vi"("error in (no error)"=w407, "Data"=w402, "Excel in"=w408) -> ()  [unwired: 7 in, 2 out]
        }
        frame "Refresh" {
          n238 = Unbundle By Name(w443) -> ("Refresh"=w442:refnum<vi>)
          n239 = property class="Bool (strict)"(reference=w442) -> (reference out=w440:refnum<vi>, error out=w444:errorcluster, "Value"=w446:bool)  [unwired: 1 in]
          n240 = Variant To Data(error in=w444, type=TRUE, Variant=w446) -> (data=w441:bool, error out=w438:errorcluster)
          n241 = call <vilib>:"Clear Errors.vi"("error in (no error)"=w438) -> ()  [unwired: 5 in, 2 out]
          n242 = case shown="True" w441 {
            tunnel: w448 -> [_ w453]
            tunnel: w440 -> [w450 w451]
            tunnel: [w450 w451] -> w439
            frame False {
            }
            frame True {
              w452 = T2[] [enum."Copy data", enum."Perform FFT", enum."Update cursors"] items=["Initialise", "Copy data", "Update cursors", "Perform FFT", "Launch inspection window", "Write to Excel", "Refresh", "Exit"]
              n243 = Enqueue Element(queue=w453, element=w452) -> ()  [unwired: 2 in, 3 out]
            }
          }
          n244 = property class="Bool (strict)"(reference=w439, "Value"=FALSE) -> (error out=w437:errorcluster)  [unwired: 1 in, 1 out]
          n245 = call <vilib>:"Clear Errors.vi"("error in (no error)"=w437) -> ()  [unwired: 5 in, 2 out]
        }
        frame "Exit" {
          (unwired) TRUE
          # "Stop GUI Loop"
          n246 = property on="stop" class="Bool (strict)"("Val(Sgnl)"=TRUE ("Value (Signaling)")) -> ()  [unwired: 2 in, 2 out]
          n247 = local write "Abort"(TRUE ("stop")) -> ()
          n248 = control-ref of="This VI"() -> (w457:refnum<vi>)
        }
      }
    }
  }
  n249 = Not A Number/Path/Refnum?(number/path/refnum="Centre VI") -> (NaN/Path/Refnum?=w5:bool)
  n250 = Not(x=w5) -> (.not. x?=w4:bool)
  n251 = call <userlib>:"Is Executable.vi"() -> ("exe?"=w3:bool)  [unwired: 5 in]
  n252 = Or(x=w3, y=w4) -> (x .or. y?=w2:bool)
  n253 = case shown="True" w2 {
    tunnel: w12 -> [_ w461]
    frame False {
    }
    frame True {
      n254 = property class="VI"(reference=w461, "FP.State"=T8."Closed" ("Front Panel Window:State")) -> (error out=w459:errorcluster)  [unwired: 1 in, 1 out]
      n255 = call <vilib>:"Clear Errors.vi"("error in (no error)"=w459) -> ()  [unwired: 5 in, 2 out]
    }
  }
